vi "IV(H)_2devices_DC_vector_magnet_stable+sweep_BF_LD-400_K6221_K2182A_PK.vi"() -> ()   [LabVIEW 2016]
uses:
  Labview Drivers/Keithley 622x LV 2009/Keithley 622x.lvlib
  Labview Drivers/lake_shore_372/Lake Shore 372/Lake Shore 372.lvlib
panel:
  out "Still temperature (K)":dbl=0.747234 min=0.0 max=1000.0 step=1e-05 format="%^.5e"
  out "Still Output (%)":dbl=13.69 min=0.0 max=100.0 step=1e-05 format="%^.5e"
  out "Magnet temperature (K)":dbl=3.7122 min=0.0 max=1000.0 step=1e-05 format="%.5f"
  in  "From 5":dbl[](array[numeric])=[0.0] min=-3000.0 max=3000.0 format="%#.5f"
  in  "To 5":dbl[](array[numeric])=[0.0] min=-3000.0 max=3000.0 format="%#.5g"
  in  "Step 5":dbl[](array[numeric])=[0.001] min=-3000.0 max=3000.0 format="%.5e"
  in  "Still Heater Output (%)":dbl=13.69
  in  "Heater Range (0: Off)":u16(ring)=6 items=["Off", "31.6 uA", "100 uA", "316 uA", "1.00 mA", "3.16 mA", "10.0 mA", "31.6 mA", "100 mA"]
  in  "Output (0: sample heater)":u16(ring) items=["sample heater", "output 1 (warm-up heater) ", "output 2 (analog/still)"]
  in  "Rate(D) (0)":dbl min=0.0 max=2500.0 step=1.0 format="%.6f"
  in  "Reset(I) (20)":dbl=20.0 min=0.0 max=10000.0 step=1.0 format="%.6f"
  in  "Gain(P) (10.000)":dbl=10.0 min=0.001 max=1000.0 step=0.001 format="%.6f"
  out "Set Temperature (K)":dbl=0.9999999999999999 format="%#_13g"
  out "Delay timer (s)":i32=600
  in  "T settling delay (s)":i32=60
  out "Heater Output (%)":dbl=7.0 min=0.0 max=100.0 step=1e-05 format="%^.5e"
  out "Current Temperature (K)":dbl=1.00279 format="%#_13g"
  out "data 2":dbl[](array[numeric])=[0.0, 0.1539956170131437, 179.99925141305565, -5.8e-05, -0.000894677769, 15.42547877586207, 62218.001]
  out "File path 2":path=path "D:/Malli/GeTe/VNM519/027_VNM519_Dev1_DC_IV_baseT_OOP-Y-axis(250_to_-250mT)_1mT_steps_I16-19_V17-18_(K6221_12- K2182_4).dat"
  in  "Measure two devices?":bool
  in  "Number Averaging":i32=1
  in  "Tab Control":enum32{"Device 1", "Device 2"}(tab)
  out "V vs I":cluster{dbl, "Field Reading":dbl}[](graph)=[{0.0, "Field Reading"=-1.52268497e-07}, {2e-07, "Field Reading"=-7.97594228e-08}, {4e-07, "Field Reading"=-2.74494669e-08}, {6e-07, "Field Reading"=2.5999633e-07}, {8e-07, "Field Reading"=6.6863549e-07}, {1e-06, "Field Reading"=9.26042323e-07}, {1.2e-06, "Field Reading"=1.14823021e-06}, {1.4e-06, "Field Reading"=1.4843606e-06}, {1.6e-06, "Field Reading"=1.76714547e-06}, {1.8e-06, "Field Reading"=1.96654487e-06}, {2e-06, "Field Reading"=2.31562332e-06}, {2.2e-06, "Field Reading"=2.42801356e-06}, {2.4e-06, "Field Reading"=2.6657392e-06}, {2.6e-06, "Field Reading"=3.04123176e-06}, {2.8e-06, "Field Reading"=3.30122805e-06}, {3e-06, "Field Reading"=3.42190359e-06}, {3.2e-06, "Field Reading"=3.80050368e-06}, {3.4e-06, "Field Reading"=3.8305433e-06}, {3.6e-06, "Field Reading"=4.18790866e-06}, {3.8e-06, "Field Reading"=4.36969886e-06}, {4e-06, "Field Reading"=4.7099712e-06}, {4.2e-06, "Field Reading"=5.08080239e-06}, {4.4e-06, "Field Reading"=5.22633809e-06}, {4.6e-06, "Field Reading"=5.43764972e-06}, {4.8e-06, "Field Reading"=5.58784671e-06}, {5e-06, "Field Reading"=5.92760266e-06}, {5.2e-06, "Field Reading"=6.16066695e-06}, {5.4e-06, "Field Reading"=6.52631866e-06}, {5.6e-06, "Field Reading"=6.60711428e-06}, {5.8e-06, "Field Reading"=6.8862735e-06}, {6e-06, "Field Reading"=7.20945277e-06}, {6.2e-06, "Field Reading"=7.31976981e-06}, {6.4e-06, "Field Reading"=7.68645747e-06}, {6.6e-06, "Field Reading"=7.9987682e-06}, {6.8e-06, "Field Reading"=8.25462103e-06}, {7e-06, "Field Reading"=8.2913934e-06}, {7.2e-06, "Field Reading"=8.71400919e-06}, {7.4e-06, "Field Reading"=8.98850694e-06}, {7.6e-06, "Field Reading"=9.18531665e-06}, {7.8e-06, "Field Reading"=9.47948819e-06}, {8e-06, "Field Reading"=9.61984449e-06}, {8.2e-06, "Field Reading"=9.91195133e-06}, {8.4e-06, "Field Reading"=1.00347079e-05}, {8.6e-06, "Field Reading"=1.03490855e-05}, {8.8e-06, "Field Reading"=1.06489614e-05}, {9e-06, "Field Reading"=1.08991132e-05}, {9.2e-06, "Field Reading"=1.1134249e-05}, {9.4e-06, "Field Reading"=1.13165569e-05}, {9.6e-06, "Field Reading"=1.15257967e-05}, {9.8e-06, "Field Reading"=1.18443188e-05}, {1e-05, "Field Reading"=1.21214061e-05}, {1.02e-05, "Field Reading"=1.23254667e-05}, {1.04e-05, "Field Reading"=1.26320829e-05}, {1.06e-05, "Field Reading"=1.27895307e-05}, {1.08e-05, "Field Reading"=1.30749049e-05}, {1.1e-05, "Field Reading"=1.32494289e-05}, {1.12e-05, "Field Reading"=1.34664374e-05}, {1.14e-05, "Field Reading"=1.3915992e-05}, {1.16e-05, "Field Reading"=1.40470318e-05}, {1.18e-05, "Field Reading"=1.43101353e-05}, {1.2e-05, "Field Reading"=1.45571832e-05}, {1.22e-05, "Field Reading"=1.46328053e-05}, {1.24e-05, "Field Reading"=1.50393728e-05}, {1.26e-05, "Field Reading"=1.51921593e-05}, {1.28e-05, "Field Reading"=1.54972138e-05}, {1.3e-05, "Field Reading"=1.57333855e-05}, {1.32e-05, "Field Reading"=1.59866486e-05}, {1.34e-05, "Field Reading"=1.6305696e-05}, {1.36e-05, "Field Reading"=1.64346582e-05}, {1.38e-05, "Field Reading"=1.66801526e-05}, {1.4e-05, "Field Reading"=1.69613835e-05}, {1.42e-05, "Field Reading"=1.71208941e-05}, {1.44e-05, "Field Reading"=1.74218058e-05}, {1.46e-05, "Field Reading"=1.76522803e-05}, {1.48e-05, "Field Reading"=1.80106844e-05}, {1.5e-05, "Field Reading"=1.80904442e-05}, {1.52e-05, "Field Reading"=1.83623524e-05}, {1.54e-05, "Field Reading"=1.86627412e-05}, {1.56e-05, "Field Reading"=1.88631763e-05}, {1.58e-05, "Field Reading"=1.90320183e-05}, {1.6e-05, "Field Reading"=1.93800576e-05}, {1.62e-05, "Field Reading"=1.9578939e-05}, {1.64e-05, "Field Reading"=1.97788562e-05}, {1.66e-05, "Field Reading"=2.00880632e-05}, {1.68e-05, "Field Reading"=2.0350131e-05}, {1.7e-05, "Field Reading"=2.05593708e-05}, {1.72e-05, "Field Reading"=2.0896531e-05}, {1.74e-05, "Field Reading"=2.10658909e-05}, {1.76e-05, "Field Reading"=2.11917455e-05}, {1.78e-05, "Field Reading"=2.15387632e-05}, {1.8e-05, "Field Reading"=2.17775246e-05}, {1.82e-05, "Field Reading"=2.19841749e-05}, {1.84e-05, "Field Reading"=2.22824971e-05}, {1.86e-05, "Field Reading"=2.24321761e-05}, {1.88e-05, "Field Reading"=2.27020127e-05}, {1.9e-05, "Field Reading"=2.29822077e-05}, {1.92e-05, "Field Reading"=2.32157907e-05}, {1.94e-05, "Field Reading"=2.3448855e-05}, {1.96e-05, "Field Reading"=2.36135537e-05}, {1.98e-05, "Field Reading"=2.38725181e-05}, {2e-05, "Field Reading"=2.41837884e-05}, {2.02e-05, "Field Reading"=2.43945821e-05}, {2.04e-05, "Field Reading"=2.46193413e-05}, {2.06e-05, "Field Reading"=2.49093766e-05}, {2.08e-05, "Field Reading"=2.51222418e-05}, {2.1e-05, "Field Reading"=2.52900611e-05}, {2.12e-05, "Field Reading"=2.55407347e-05}, {2.14e-05, "Field Reading"=2.58758293e-05}, {2.16e-05, "Field Reading"=2.60860873e-05}, {2.18e-05, "Field Reading"=2.6178795e-05}, {2.2e-05, "Field Reading"=2.6620063e-05}, {2.22e-05, "Field Reading"=2.67676686e-05}, {2.24e-05, "Field Reading"=2.69230447e-05}, {2.26e-05, "Field Reading"=2.72975009e-05}, {2.28e-05, "Field Reading"=2.7582357e-05}, {2.3e-05, "Field Reading"=2.77507011e-05}, {2.32e-05, "Field Reading"=2.80096614e-05}, {2.34e-05, "Field Reading"=2.81696988e-05}, {2.36e-05, "Field Reading"=2.85907685e-05}, {2.38e-05, "Field Reading"=2.87735944e-05}, {2.4e-05, "Field Reading"=2.90294472e-05}, {2.42e-05, "Field Reading"=2.9178615e-05}, {2.44e-05, "Field Reading"=2.96002024e-05}, {2.46e-05, "Field Reading"=2.9786136e-05}, {2.48e-05, "Field Reading"=2.99565396e-05}, {2.6e-05, "Field Reading"=3.14186299e-05}, {2.7e-05, "Field Reading"=3.26751057e-05}, {2.8e-05, "Field Reading"=3.38378258e-05}, {2.9e-05, "Field Reading"=3.52035824e-05}, {3e-05, "Field Reading"=3.63435256e-05}, {3e-05, "Field Reading"=3.63673343e-05}, {1.501e-05, "Field Reading"=1.79573366e-05}, {2e-08, "Field Reading"=-3.87921991e-07}, {0.0, "Field Reading"=-3.45452353e-07}, {-2e-07, "Field Reading"=-3.83778479e-07}, {-4e-07, "Field Reading"=-4.92023888e-07}, {-6e-07, "Field Reading"=-7.5460964e-07}, {-8e-07, "Field Reading"=-1.24196958e-06}, {-1e-06, "Field Reading"=-1.538736e-06}, {-1.2e-06, "Field Reading"=-1.68893191e-06}, {-1.4e-06, "Field Reading"=-2.02972104e-06}, {-1.6e-06, "Field Reading"=-2.24103112e-06}, {-1.8e-06, "Field Reading"=-2.59114291e-06}, {-2e-06, "Field Reading"=-2.7993462e-06}, {-2.2e-06, "Field Reading"=-2.92209253e-06}, {-2.4e-06, "Field Reading"=-3.30068989e-06}, {-2.6e-06, "Field Reading"=-3.44466872e-06}, {-2.8e-06, "Field Reading"=-3.70673454e-06}, {-3e-06, "Field Reading"=-3.97190785e-06}, {-3.2e-06, "Field Reading"=-4.17493005e-06}, {-3.4e-06, "Field Reading"=-4.41472537e-06}, {-3.6e-06, "Field Reading"=-4.66177152e-06}, {-3.8e-06, "Field Reading"=-4.9191763e-06}, {-4e-06, "Field Reading"=-5.20920954e-06}, {-4.2e-06, "Field Reading"=-5.55465984e-06}, {-4.4e-06, "Field Reading"=-5.66652605e-06}, {-4.6e-06, "Field Reading"=-5.96691739e-06}, {-4.8e-06, "Field Reading"=-6.19013923e-06}, {-5e-06, "Field Reading"=-6.40818191e-06}, {-5.2e-06, "Field Reading"=-6.672842e-06}, {-5.4e-06, "Field Reading"=-6.9483736e-06}, {-5.6e-06, "Field Reading"=-7.18713312e-06}, {-5.8e-06, "Field Reading"=-7.36218605e-06}, {-6e-06, "Field Reading"=-7.68329416e-06}, {-6.2e-06, "Field Reading"=-7.86922612e-06}, {-6.4e-06, "Field Reading"=-8.26853861e-06}, {-6.6e-06, "Field Reading"=-8.30634649e-06}, {-6.8e-06, "Field Reading"=-8.59586168e-06}, {-7e-06, "Field Reading"=-9.00657456e-06}, {-7.2e-06, "Field Reading"=-9.14951953e-06}, {-7.4e-06, "Field Reading"=-9.39708366e-06}, {-7.6e-06, "Field Reading"=-9.56643916e-06}, {-7.8e-06, "Field Reading"=-9.81970027e-06}, {-8e-06, "Field Reading"=-1.00263489e-05}, {-8.2e-06, "Field Reading"=-1.02837565e-05}, {-8.4e-06, "Field Reading"=-1.06437086e-05}, {-8.6e-06, "Field Reading"=-1.07623114e-05}, {-8.8e-06, "Field Reading"=-1.09855426e-05}, {-9e-06, "Field Reading"=-1.11694032e-05}, {-9.2e-06, "Field Reading"=-1.15034596e-05}, {-9.4e-06, "Field Reading"=-1.17209848e-05}, {-9.6e-06, "Field Reading"=-1.19462748e-05}, {-9.8e-06, "Field Reading"=-1.21871062e-05}, {-1e-05, "Field Reading"=-1.24362242e-05}, {-1.02e-05, "Field Reading"=-1.26667036e-05}, {-1.04e-05, "Field Reading"=-1.30364964e-05}, {-1.06e-05, "Field Reading"=-1.32317511e-05}, {-1.08e-05, "Field Reading"=-1.35373222e-05}, {-1.1e-05, "Field Reading"=-1.37237724e-05}, {-1.12e-05, "Field Reading"=-1.40371123e-05}, {-1.14e-05, "Field Reading"=-1.42893266e-05}, {-1.16e-05, "Field Reading"=-1.43830695e-05}, {-1.18e-05, "Field Reading"=-1.46358129e-05}, {-1.2e-05, "Field Reading"=-1.50543024e-05}, {-1.22e-05, "Field Reading"=-1.51656546e-05}, {-1.24e-05, "Field Reading"=-1.54468836e-05}, {-1.26e-05, "Field Reading"=-1.56442061e-05}, {-1.28e-05, "Field Reading"=-1.580735e-05}, {-1.3e-05, "Field Reading"=-1.61113673e-05}, {-1.32e-05, "Field Reading"=-1.62418839e-05}, {-1.34e-05, "Field Reading"=-1.6634983e-05}, {-1.36e-05, "Field Reading"=-1.68178077e-05}, {-1.38e-05, "Field Reading"=-1.69198374e-05}, {-1.4e-05, "Field Reading"=-1.7212986e-05}, {-1.42e-05, "Field Reading"=-1.74341367e-05}, {-1.44e-05, "Field Reading"=-1.77231346e-05}, {-1.46e-05, "Field Reading"=-1.78510457e-05}, {-1.48e-05, "Field Reading"=-1.81830304e-05}, {-1.5e-05, "Field Reading"=-1.83668909e-05}, {-1.52e-05, "Field Reading"=-1.86812606e-05}, {-1.54e-05, "Field Reading"=-1.87755215e-05}, {-1.56e-05, "Field Reading"=-1.91867473e-05}, {-1.58e-05, "Field Reading"=-1.92447572e-05}, {-1.6e-05, "Field Reading"=-1.95373802e-05}, {-1.62e-05, "Field Reading"=-1.98776515e-05}, {-1.64e-05, "Field Reading"=-2.01619878e-05}, {-1.66e-05, "Field Reading"=-2.03448124e-05}, {-1.68e-05, "Field Reading"=-2.05985916e-05}, {-1.7e-05, "Field Reading"=-2.09740769e-05}, {-1.72e-05, "Field Reading"=-2.10243148e-05}, {-1.74e-05, "Field Reading"=-2.14578111e-05}, {-1.76e-05, "Field Reading"=-2.17752926e-05}, {-1.78e-05, "Field Reading"=-2.20503063e-05}, {-1.8e-05, "Field Reading"=-2.21507822e-05}, {-1.82e-05, "Field Reading"=-2.23900597e-05}, {-1.84e-05, "Field Reading"=-2.26723233e-05}, {-1.86e-05, "Field Reading"=-2.28976171e-05}, {-1.88e-05, "Field Reading"=-2.31016762e-05}, {-1.9e-05, "Field Reading"=-2.34289957e-05}, {-1.92e-05, "Field Reading"=-2.37117782e-05}, {-1.94e-05, "Field Reading"=-2.40458343e-05}, {-1.96e-05, "Field Reading"=-2.40541191e-05}, {-1.98e-05, "Field Reading"=-2.44544686e-05}, {-2e-05, "Field Reading"=-2.46621531e-05}, {-2.02e-05, "Field Reading"=-2.49703066e-05}, {-2.04e-05, "Field Reading"=-2.5097714e-05}, {-2.06e-05, "Field Reading"=-2.54835617e-05}, {-2.08e-05, "Field Reading"=-2.55648796e-05}, {-2.1e-05, "Field Reading"=-2.58497336e-05}, {-2.12e-05, "Field Reading"=-2.60413627e-05}, {-2.14e-05, "Field Reading"=-2.64365387e-05}, {-2.16e-05, "Field Reading"=-2.67032657e-05}, {-2.18e-05, "Field Reading"=-2.68964486e-05}, {-2.2e-05, "Field Reading"=-2.71341792e-05}, {-2.22e-05, "Field Reading"=-2.72719451e-05}, {-2.24e-05, "Field Reading"=-2.75303855e-05}, {-2.26e-05, "Field Reading"=-2.79266128e-05}, {-2.28e-05, "Field Reading"=-2.81301542e-05}, {-2.3e-05, "Field Reading"=-2.83901486e-05}, {-2.32e-05, "Field Reading"=-2.84232953e-05}, {-2.34e-05, "Field Reading"=-2.87630526e-05}, {-2.36e-05, "Field Reading"=-2.91333634e-05}, {-2.38e-05, "Field Reading"=-2.9317224e-05}, {-2.4e-05, "Field Reading"=-2.96481828e-05}, {-2.42e-05, "Field Reading"=-2.98304898e-05}, {-2.44e-05, "Field Reading"=-2.99692916e-05}, {-2.46e-05, "Field Reading"=-3.02660647e-05}, {-2.48e-05, "Field Reading"=-3.04944663e-05}, {-2.6e-05, "Field Reading"=-3.20653099e-05}, {-2.7e-05, "Field Reading"=-3.32523697e-05}, {-2.8e-05, "Field Reading"=-3.44534201e-05}, {-2.9e-05, "Field Reading"=-3.56938321e-05}, {-3e-05, "Field Reading"=-3.69958442e-05}, {-3e-05, "Field Reading"=-3.70222579e-05}, {-1.501e-05, "Field Reading"=-1.84243803e-05}, {-2e-08, "Field Reading"=-2.59477872e-07}]
  in  "File name 1":string="011_31-05-2022_DevB4_DC_IV(H)_baseT_[5_to-5mT]_30uT_steps_(0_deg)_I_10-36_V_12-37_100nA_steps"
  in  "From 3":dbl[](array[numeric])=[0.0, 2e-05, 0.0, -2e-05] min=-3000.0 max=3000.0 format="%.1e"
  in  "To 3":dbl[](array[numeric])=[2e-05, 0.0, -2e-05, 0.0] min=-3000.0 max=3000.0 format="%.1e"
  in  "Step 3":dbl[](array[numeric])=[2e-08, 9.99e-06, 2e-08, 9.99e-06] min=-3000.0 max=3000.0 format="%.1e"
  in  "Current source K6221 VISA Device 1":refnum<visa-resource-name>="GPIB0::13::INSTR"
  in  "Nanovoltmeter 2182a VISA Device1":refnum<visa-resource-name>="GPIB0::7::INSTR"
  in  "wait (ms)":u32=50
  in  "Set Compliance voltage (V)":dbl=2.0 min=0.0 step=0.1 format="%_3f"
  out "Resistance (ohm)":dbl=12.9738936 format="%#_13g"
  out "Time (s)":dbl=151861.951 format="%#_13g"
  out "Iset (A)":dbl=-2e-08
  out "Vmeas (V)":dbl=-2.59477872e-07
  in  "File name 2":string="040_31-05-2023_DevB3_DC_IV(A)_baseT_12mT_(0-360deg)_5deg_steps_I_10-38_V_12-31_"
  in  "Current source K6221 VISA Device 2":refnum<visa-resource-name>="GPIB0::13::INSTR"
  in  "Nanovoltmeter 2182a VISA Device 2":refnum<visa-resource-name>="GPIB0::7::INSTR"
  in  "Set Compliance voltage (V) 2":dbl=2.0 min=0.0 step=0.1 format="%_3f"
  in  "wait (ms) 2":u32=50
  in  "To 4":dbl[](array[numeric])=[1e-05, 3e-05, -1e-05, -0.0001, 0.0] min=-3000.0 max=3000.0 format="%.1e"
  in  "From 4":dbl[](array[numeric])=[0.0, 1.1e-05, 3e-05, 0.0, -0.0001] min=-3000.0 max=3000.0 format="%.1e"
  in  "Step 4":dbl[](array[numeric])=[2e-07, 1e-06, 0.0, 5e-07, 9.9e-05] min=-3000.0 max=3000.0 format="%.1e"
  out "V vs I 2":cluster{dbl, "Field Reading":dbl}[](graph)=[{0.0, "Field Reading"=1.05982577e-07}, {5e-07, "Field Reading"=1.23902621e-07}, {1e-06, "Field Reading"=4.09598972e-08}, {1.5e-06, "Field Reading"=7.78233302e-08}, {2e-06, "Field Reading"=7.52633791e-08}, {2.5e-06, "Field Reading"=9.9839001e-08}, {3e-06, "Field Reading"=6.70715052e-08}, {3.5e-06, "Field Reading"=6.34878296e-08}, {4e-06, "Field Reading"=1.95069789e-07}, {4.5e-06, "Field Reading"=1.48733775e-06}, {5e-06, "Field Reading"=3.68225755e-06}, {5.5e-06, "Field Reading"=7.0056209e-06}, {6e-06, "Field Reading"=1.131355e-05}, {6.5e-06, "Field Reading"=1.67191983e-05}, {7e-06, "Field Reading"=2.2852904e-05}, {7.5e-06, "Field Reading"=2.94079847e-05}, {8e-06, "Field Reading"=3.63951874e-05}, {8.5e-06, "Field Reading"=4.35057808e-05}, {9e-06, "Field Reading"=5.09056291e-05}, {9.5e-06, "Field Reading"=5.82773365e-05}, {1e-05, "Field Reading"=6.58016184e-05}, {1.05e-05, "Field Reading"=7.33770992e-05}, {1.1e-05, "Field Reading"=8.09648681e-05}, {1.15e-05, "Field Reading"=8.87364392e-05}, {1.2e-05, "Field Reading"=9.64209746e-05}, {1.25e-05, "Field Reading"=0.000104230437}, {1.3e-05, "Field Reading"=0.000112046003}, {1.35e-05, "Field Reading"=0.000119815015}, {1.4e-05, "Field Reading"=0.000127742783}, {1.45e-05, "Field Reading"=0.000135573235}, {1.5e-05, "Field Reading"=0.000143516327}, {1.55e-05, "Field Reading"=0.000151494156}, {1.6e-05, "Field Reading"=0.000159501242}, {1.65e-05, "Field Reading"=0.000167343466}, {1.7e-05, "Field Reading"=0.000175483152}, {1.75e-05, "Field Reading"=0.000183456446}, {1.8e-05, "Field Reading"=0.000191661699}, {1.85e-05, "Field Reading"=0.000199612466}, {1.9e-05, "Field Reading"=0.000207719848}, {1.95e-05, "Field Reading"=0.000215802195}, {2e-05, "Field Reading"=0.00022388403}, {2.05e-05, "Field Reading"=0.000232062763}, {2.1e-05, "Field Reading"=0.000240102107}, {2.15e-05, "Field Reading"=0.000247269011}, {2.2e-05, "Field Reading"=0.000255929973}, {2.25e-05, "Field Reading"=0.000264142372}, {2.3e-05, "Field Reading"=0.000272170452}, {2.35e-05, "Field Reading"=0.000280406012}, {2.4e-05, "Field Reading"=0.000288539055}, {2.45e-05, "Field Reading"=0.000296639977}, {2.5e-05, "Field Reading"=0.000304956829}, {2.55e-05, "Field Reading"=0.000312984916}, {2.6e-05, "Field Reading"=0.000321277684}, {2.65e-05, "Field Reading"=0.000329427113}, {2.7e-05, "Field Reading"=0.00033774076}, {2.75e-05, "Field Reading"=0.000346032008}, {2.8e-05, "Field Reading"=0.000354167609}, {2.85e-05, "Field Reading"=0.000362498087}, {2.9e-05, "Field Reading"=0.000370754002}, {2.95e-05, "Field Reading"=0.000379070387}, {3e-05, "Field Reading"=0.000387405662}, {3.05e-05, "Field Reading"=0.000395624202}, {3.1e-05, "Field Reading"=0.000403926088}, {3.15e-05, "Field Reading"=0.00041243339}, {3.2e-05, "Field Reading"=0.000420845302}, {3.25e-05, "Field Reading"=0.000429363875}, {3.3e-05, "Field Reading"=0.000437565523}, {3.35e-05, "Field Reading"=0.000446109155}, {3.4e-05, "Field Reading"=0.000454533008}, {3.45e-05, "Field Reading"=0.000463127356}, {3.5e-05, "Field Reading"=0.000471630056}, {3.55e-05, "Field Reading"=0.000479936662}, {3.6e-05, "Field Reading"=0.000488525981}, {3.65e-05, "Field Reading"=0.000497198664}, {3.7e-05, "Field Reading"=0.000505853053}, {3.75e-05, "Field Reading"=0.000514436643}, {3.8e-05, "Field Reading"=0.000522915273}, {3.85e-05, "Field Reading"=0.000531648928}, {3.9e-05, "Field Reading"=0.000540244293}, {3.95e-05, "Field Reading"=0.000548950249}, {4e-05, "Field Reading"=0.000557677924}, {4.05e-05, "Field Reading"=0.000566248716}, {4.1e-05, "Field Reading"=0.000574937679}, {4.15e-05, "Field Reading"=0.000583695347}, {4.2e-05, "Field Reading"=0.000592494999}, {4.25e-05, "Field Reading"=0.000601192661}, {4.3e-05, "Field Reading"=0.000609976951}, {4.35e-05, "Field Reading"=0.000618619419}, {4.4e-05, "Field Reading"=0.000627518275}, {4.45e-05, "Field Reading"=0.000636379362}, {4.5e-05, "Field Reading"=0.000644912509}, {4.55e-05, "Field Reading"=0.00065393999}, {4.6e-05, "Field Reading"=0.000662870466}, {4.65e-05, "Field Reading"=0.000671738209}, {4.7e-05, "Field Reading"=0.000680896763}, {4.75e-05, "Field Reading"=0.000689596876}, {4.8e-05, "Field Reading"=0.000698582898}, {4.85e-05, "Field Reading"=0.000707876118}, {4.9e-05, "Field Reading"=0.00071700519}, {4.95e-05, "Field Reading"=0.00072625694}, {5e-05, "Field Reading"=0.000735252693}, {5.05e-05, "Field Reading"=0.000744563505}, {5.1e-05, "Field Reading"=0.000753877714}, {5.15e-05, "Field Reading"=0.000763235462}, {5.2e-05, "Field Reading"=0.000772666405}, {5.25e-05, "Field Reading"=0.000781939653}, {5.3e-05, "Field Reading"=0.00079146705}, {5.35e-05, "Field Reading"=0.000801081283}, {5.4e-05, "Field Reading"=0.000810671964}, {5.45e-05, "Field Reading"=0.000820330099}, {5.5e-05, "Field Reading"=0.000830001161}, {5.55e-05, "Field Reading"=0.000839830429}, {5.6e-05, "Field Reading"=0.000849894446}, {5.65e-05, "Field Reading"=0.000859963842}, {5.7e-05, "Field Reading"=0.00087027569}, {5.75e-05, "Field Reading"=0.000880684023}, {5.8e-05, "Field Reading"=0.000891300225}, {5.85e-05, "Field Reading"=0.000901884572}, {5.9e-05, "Field Reading"=0.00091264413}, {5.95e-05, "Field Reading"=0.000923292586}, {6e-05, "Field Reading"=0.000933904184}, {6.05e-05, "Field Reading"=0.000944740541}, {6.1e-05, "Field Reading"=0.000955724863}, {6.15e-05, "Field Reading"=0.000966541693}, {6.2e-05, "Field Reading"=0.000977790203}, {6.25e-05, "Field Reading"=0.0009887668}, {6.3e-05, "Field Reading"=0.00100003886}, {6.35e-05, "Field Reading"=0.00101126331}, {6.4e-05, "Field Reading"=0.00102284095}, {6.45e-05, "Field Reading"=0.00103437413}, {6.5e-05, "Field Reading"=0.00104578697}, {6.55e-05, "Field Reading"=0.00105781627}, {6.6e-05, "Field Reading"=0.00106970781}, {6.65e-05, "Field Reading"=0.00108158658}, {6.7e-05, "Field Reading"=0.00109345152}, {6.75e-05, "Field Reading"=0.00110520407}, {6.8e-05, "Field Reading"=0.00111705365}, {6.85e-05, "Field Reading"=0.00112896007}, {6.9e-05, "Field Reading"=0.00114097245}, {6.95e-05, "Field Reading"=0.00115300225}, {7e-05, "Field Reading"=0.00116490713}, {7.05e-05, "Field Reading"=0.00117701585}, {7.1e-05, "Field Reading"=0.0011890902}, {7.15e-05, "Field Reading"=0.00120116737}, {7.2e-05, "Field Reading"=0.00121302054}, {7.25e-05, "Field Reading"=0.00122527818}, {7.3e-05, "Field Reading"=0.00123750597}, {7.35e-05, "Field Reading"=0.00124952144}, {7.4e-05, "Field Reading"=0.00126179393}, {7.45e-05, "Field Reading"=0.00127385138}, {7.5e-05, "Field Reading"=0.00128607011}, {7.55e-05, "Field Reading"=0.00129831901}, {7.6e-05, "Field Reading"=0.00131059815}, {7.65e-05, "Field Reading"=0.00132285322}, {7.7e-05, "Field Reading"=0.00133496366}, {7.75e-05, "Field Reading"=0.00134726123}, {7.8e-05, "Field Reading"=0.00135956111}, {7.85e-05, "Field Reading"=0.00137195033}, {7.9e-05, "Field Reading"=0.00138423407}, {7.95e-05, "Field Reading"=0.00139647286}, {8e-05, "Field Reading"=0.00140887898}, {8.05e-05, "Field Reading"=0.00142125669}, {8.1e-05, "Field Reading"=0.00143369762}, {8.15e-05, "Field Reading"=0.00144604179}, {8.2e-05, "Field Reading"=0.00145820055}, {8.25e-05, "Field Reading"=0.0014708299}, {8.3e-05, "Field Reading"=0.001483259}, {8.35e-05, "Field Reading"=0.00149571273}, {8.4e-05, "Field Reading"=0.00150827449}, {8.45e-05, "Field Reading"=0.00152058173}, {8.5e-05, "Field Reading"=0.00153315169}, {8.55e-05, "Field Reading"=0.00154567403}, {8.6e-05, "Field Reading"=0.00155821094}, {8.65e-05, "Field Reading"=0.00157085359}, {8.7e-05, "Field Reading"=0.00158327521}, {8.75e-05, "Field Reading"=0.00159591991}, {8.8e-05, "Field Reading"=0.00160856665}, {8.85e-05, "Field Reading"=0.00162121374}, {8.9e-05, "Field Reading"=0.00163385997}, {8.95e-05, "Field Reading"=0.00164634288}, {9e-05, "Field Reading"=0.00165906267}, {9.05e-05, "Field Reading"=0.00167177904}, {9.1e-05, "Field Reading"=0.00168450438}, {9.15e-05, "Field Reading"=0.00169730779}, {9.2e-05, "Field Reading"=0.00170982705}, {9.25e-05, "Field Reading"=0.00172262613}, {9.3e-05, "Field Reading"=0.00173539114}, {9.35e-05, "Field Reading"=0.00174822988}, {9.4e-05, "Field Reading"=0.00176107221}, {9.45e-05, "Field Reading"=0.00177372408}, {9.5e-05, "Field Reading"=0.00178659463}, {9.55e-05, "Field Reading"=0.00179942159}, {9.6e-05, "Field Reading"=0.00181213335}, {9.65e-05, "Field Reading"=0.00182507038}, {9.7e-05, "Field Reading"=0.00183795264}, {9.75e-05, "Field Reading"=0.00185079437}, {9.8e-05, "Field Reading"=0.0018638159}, {9.85e-05, "Field Reading"=0.00187644421}, {9.9e-05, "Field Reading"=0.0018893681}, {9.95e-05, "Field Reading"=0.001902598}, {0.0001, "Field Reading"=0.00191566643}, {0.0001, "Field Reading"=0.00191578214}, {1e-06, "Field Reading"=1.04959382e-07}, {0.0, "Field Reading"=6.2978119e-08}, {-5e-07, "Field Reading"=7.37299411e-08}, {-1e-06, "Field Reading"=7.32183306e-08}, {-1.5e-06, "Field Reading"=9.8305911e-08}, {-2e-06, "Field Reading"=9.8305911e-08}, {-2.5e-06, "Field Reading"=-9.212857e-09}, {-3e-06, "Field Reading"=7.52657514e-08}, {-3.5e-06, "Field Reading"=-2.29881222e-07}, {-4e-06, "Field Reading"=-9.66638942e-07}, {-4.5e-06, "Field Reading"=-2.71867509e-06}, {-5e-06, "Field Reading"=-5.44042382e-06}, {-5.5e-06, "Field Reading"=-9.24299578e-06}, {-6e-06, "Field Reading"=-1.39195329e-05}, {-6.5e-06, "Field Reading"=-1.93947706e-05}, {-7e-06, "Field Reading"=-2.53845658e-05}, {-7.5e-06, "Field Reading"=-3.17772987e-05}, {-8e-06, "Field Reading"=-3.85647725e-05}, {-8.5e-06, "Field Reading"=-4.54935603e-05}, {-9e-06, "Field Reading"=-5.25713378e-05}, {-9.5e-06, "Field Reading"=-5.9848778e-05}, {-1e-05, "Field Reading"=-6.72593486e-05}, {-1.05e-05, "Field Reading"=-7.46959979e-05}, {-1.1e-05, "Field Reading"=-8.22145956e-05}, {-1.15e-05, "Field Reading"=-8.98888387e-05}, {-1.2e-05, "Field Reading"=-9.7508345e-05}, {-1.25e-05, "Field Reading"=-0.000105279358}, {-1.3e-05, "Field Reading"=-0.000112994564}, {-1.35e-05, "Field Reading"=-0.000120810121}, {-1.4e-05, "Field Reading"=-0.000128620045}, {-1.45e-05, "Field Reading"=-0.00013646688}, {-1.5e-05, "Field Reading"=-0.000144369477}, {-1.55e-05, "Field Reading"=-0.000152356042}, {-1.6e-05, "Field Reading"=-0.00016028334}, {-1.65e-05, "Field Reading"=-0.000168222807}, {-1.7e-05, "Field Reading"=-0.000176283573}, {-1.75e-05, "Field Reading"=-0.000184271677}, {-1.8e-05, "Field Reading"=-0.000192294085}, {-1.85e-05, "Field Reading"=-0.000200345666}, {-1.9e-05, "Field Reading"=-0.00020833633}, {-1.95e-05, "Field Reading"=-0.000216423693}, {-2e-05, "Field Reading"=-0.000224573584}, {-2.05e-05, "Field Reading"=-0.000232658964}, {-2.1e-05, "Field Reading"=-0.000240789835}, {-2.15e-05, "Field Reading"=-0.00024942458}, {-2.2e-05, "Field Reading"=-0.000257524758}, {-2.25e-05, "Field Reading"=-0.000265682837}, {-2.3e-05, "Field Reading"=-0.000273921299}, {-2.35e-05, "Field Reading"=-0.000281918732}, {-2.4e-05, "Field Reading"=-0.000290019983}, {-2.45e-05, "Field Reading"=-0.000298346441}, {-2.5e-05, "Field Reading"=-0.000306562888}, {-2.55e-05, "Field Reading"=-0.000314745032}, {-2.6e-05, "Field Reading"=-0.000322866101}, {-2.65e-05, "Field Reading"=-0.000331147056}, {-2.7e-05, "Field Reading"=-0.000339239598}, {-2.75e-05, "Field Reading"=-0.000347604575}, {-2.8e-05, "Field Reading"=-0.000355902938}, {-2.85e-05, "Field Reading"=-0.000364053667}, {-2.9e-05, "Field Reading"=-0.000372274716}, {-2.95e-05, "Field Reading"=-0.000380721042}, {-3e-05, "Field Reading"=-0.000389052226}, {-3.05e-05, "Field Reading"=-0.000397248701}, {-3.1e-05, "Field Reading"=-0.000405627052}, {-3.15e-05, "Field Reading"=-0.000414022694}, {-3.2e-05, "Field Reading"=-0.000422452566}, {-3.25e-05, "Field Reading"=-0.000430871246}, {-3.3e-05, "Field Reading"=-0.000439115251}, {-3.35e-05, "Field Reading"=-0.000447710054}, {-3.4e-05, "Field Reading"=-0.000456261339}, {-3.45e-05, "Field Reading"=-0.000464751635}, {-3.5e-05, "Field Reading"=-0.000473286534}, {-3.55e-05, "Field Reading"=-0.00048171494}, {-3.6e-05, "Field Reading"=-0.000490283148}, {-3.65e-05, "Field Reading"=-0.000498827776}, {-3.7e-05, "Field Reading"=-0.000507439986}, {-3.75e-05, "Field Reading"=-0.000516045781}, {-3.8e-05, "Field Reading"=-0.0005246155}, {-3.85e-05, "Field Reading"=-0.000533221482}, {-3.9e-05, "Field Reading"=-0.000541909479}, {-3.95e-05, "Field Reading"=-0.000550577507}, {-4e-05, "Field Reading"=-0.000559311386}, {-4.05e-05, "Field Reading"=-0.000567846814}, {-4.1e-05, "Field Reading"=-0.00057664276}, {-4.15e-05, "Field Reading"=-0.000585338952}, {-4.2e-05, "Field Reading"=-0.000594088391}, {-4.25e-05, "Field Reading"=-0.00060273111}, {-4.3e-05, "Field Reading"=-0.000611546081}, {-4.35e-05, "Field Reading"=-0.00062030934}, {-4.4e-05, "Field Reading"=-0.000629159621}, {-4.45e-05, "Field Reading"=-0.0006379664}, {-4.5e-05, "Field Reading"=-0.000646666684}, {-4.55e-05, "Field Reading"=-0.000655509687}, {-4.6e-05, "Field Reading"=-0.000664396847}, {-4.65e-05, "Field Reading"=-0.000673287336}, {-4.7e-05, "Field Reading"=-0.000682299425}, {-4.75e-05, "Field Reading"=-0.000691233691}, {-4.8e-05, "Field Reading"=-0.000700295086}, {-4.85e-05, "Field Reading"=-0.00070939524}, {-4.9e-05, "Field Reading"=-0.000718437027}, {-4.95e-05, "Field Reading"=-0.000727632333}, {-5e-05, "Field Reading"=-0.000736695622}, {-5.05e-05, "Field Reading"=-0.000746025716}, {-5.1e-05, "Field Reading"=-0.000755243116}, {-5.15e-05, "Field Reading"=-0.000764786655}, {-5.2e-05, "Field Reading"=-0.000774240444}, {-5.25e-05, "Field Reading"=-0.000783658543}, {-5.3e-05, "Field Reading"=-0.000793342878}, {-5.35e-05, "Field Reading"=-0.000803049948}, {-5.4e-05, "Field Reading"=-0.000812865349}, {-5.45e-05, "Field Reading"=-0.000822671023}, {-5.5e-05, "Field Reading"=-0.000832792343}, {-5.55e-05, "Field Reading"=-0.000842879097}, {-5.6e-05, "Field Reading"=-0.000853268375}, {-5.65e-05, "Field Reading"=-0.000863553781}, {-5.7e-05, "Field Reading"=-0.00087382946}, {-5.75e-05, "Field Reading"=-0.000884019633}, {-5.8e-05, "Field Reading"=-0.000894677769}]
  out "Vmeas (V) 2":dbl=-0.000894677769
  out "Resistance (ohm) 2":dbl=15.42547877586207 format="%#_13g"
  out "Iset (A) 2":dbl=-5.8e-05
  out "Sweeping Magnetic Field magnitude(T)":dbl=284.9997059221995 format="%#_13g"
  out "Stable Magnetic Field magnitude (T)":dbl=0.11799861557435369 format="%#_13g"
  in  "From 2":dbl[](array[numeric])=[0.005] min=-3000.0 max=3000.0 format="%#.5f"
  in  "To 2":dbl[](array[numeric])=[-0.005] min=-3000.0 max=3000.0 format="%#.5g"
  in  "Step 2":dbl[](array[numeric])=[3e-05] min=-3000.0 max=3000.0 format="%.5e"
  in  "Wait time after each sweep(min)":dbl=0.1 format="%#_13g"
  in  "Sweep Field ramp rate (T/min)":string="0.0005"
  in  "Stable Field ramp rate (T/min)":string="0.0005"
  in  "Magnet IP Address \n(Stable field)":string="169.254.207.70"
  in  "Magnet IP Address\n(Sweeping  field)":string="169.254.67.34"
  in  "Magnetic field stabilization time (s)":dbl=1.0 format="%#_13g"
  in  "Step":dbl[](array[numeric])=[0.001] min=-3000.0 max=3000.0 format="%.4g"
  in  "To":dbl[](array[numeric])=[0.0] min=-3000.0 max=3000.0 format="%.4f"
  in  "From":dbl[](array[numeric])=[0.0] min=-3000.0 max=3000.0 format="%.4f"
  in  "Folder":path=path "D:/Pranava/Data/PtTe2/31-05-2022/001/Round8_IP/after warmup"
  out "data":dbl[](array[numeric])=[1.00279, 0.11799861557435369, 284.9997059221995, -2e-08, -2.59477872e-07, 12.9738936, 151861.951]
  out "File path 1":path=path "D:/Pranava/Data/PtTe2/31-05-2022/001/Round8_IP/after warmup/011_31-05-2022_DevB4_DC_IV(H)_baseT_[5_to-5mT]_30uT_steps_(0_deg)_I_10-36_V_12-37_100nA_steps.dat"
  # "11.5% corresponds to 7mW\n13.69% corresponds to 10mW\nSet to 0 if you want to use at 1K"
  # "[Must be less than 0.05]"
  # "It is important that there is enough time for the magnet to cool down after each sweep (Typically 15-20 min)"
  # "Configure Temperature (K)"
  # "Configure Stable Field (T)"
  # "Configure Sweeping Field(T)"
  # "Z-Axis: In-plane (90 deg)\nY-axis: Out-of-plane (0 deg)"
  # ".dat"
  # "Configure current sweep 1 (A)"
  # ".dat"
  # "Configure current sweep 2 (A)"
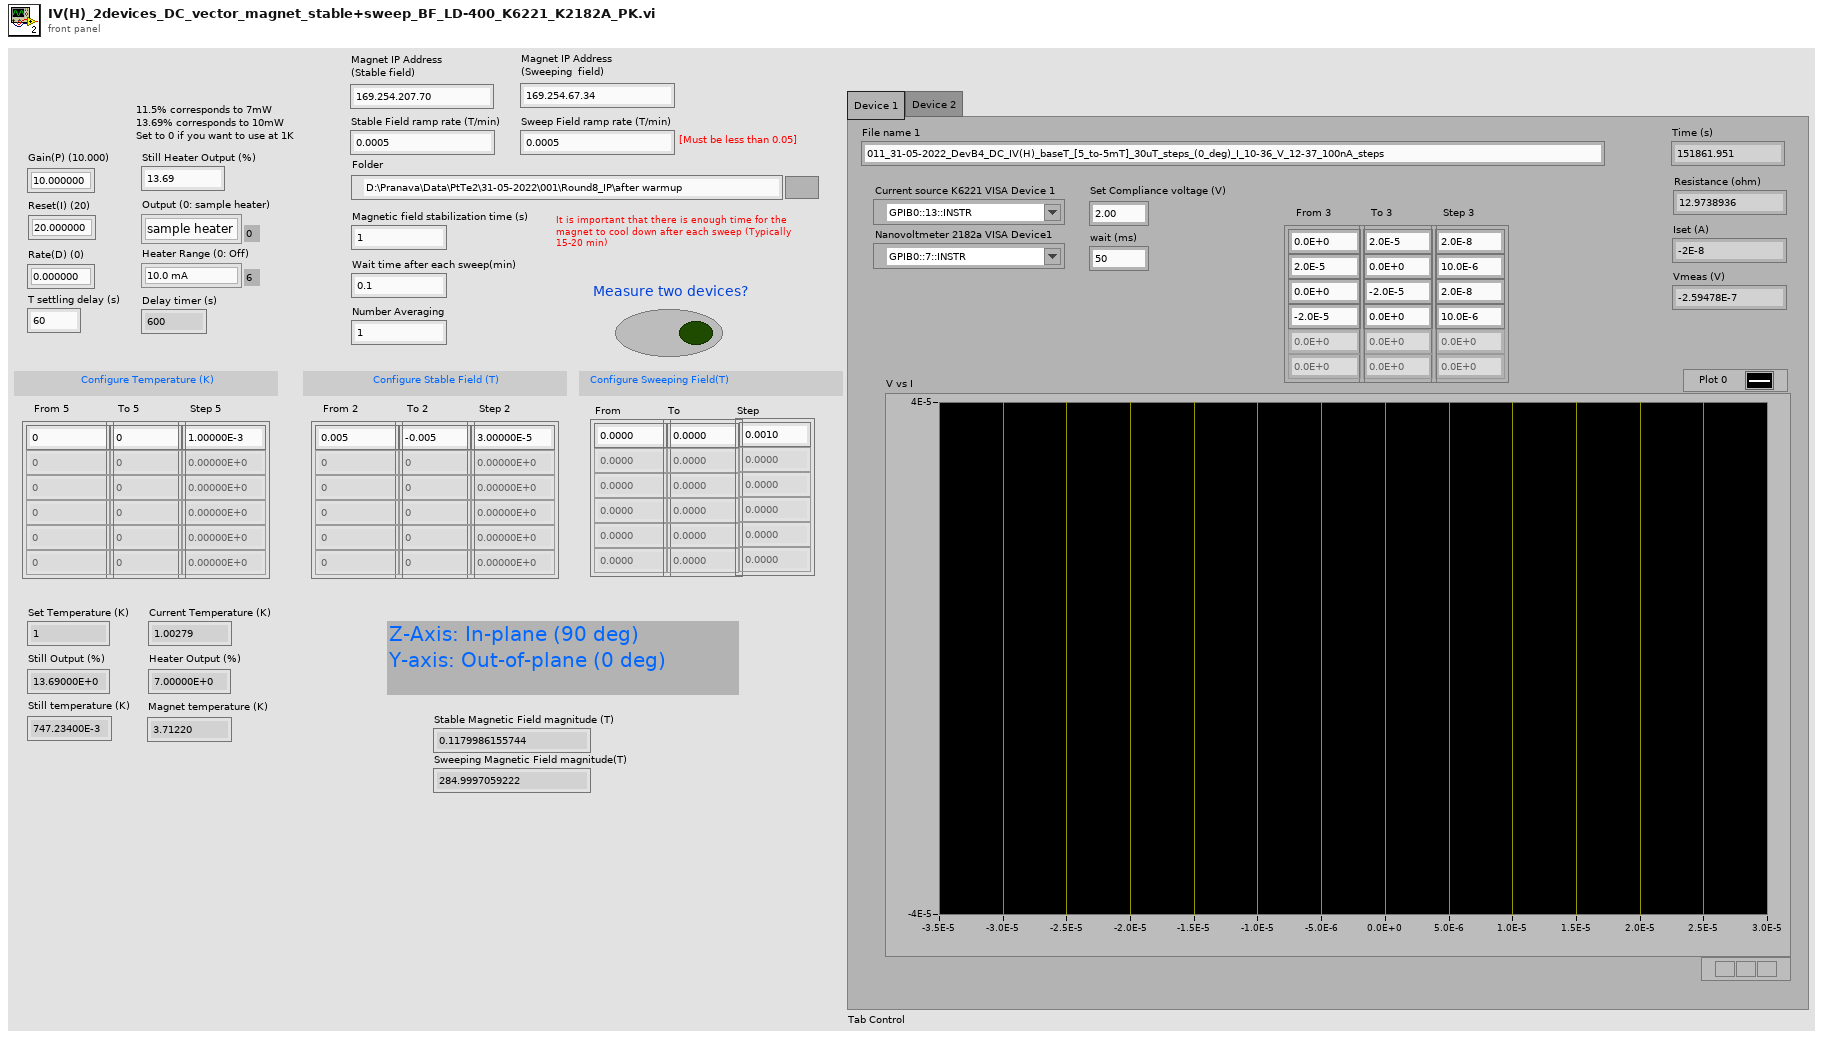
[diagram p1: front panel]
types:
  T1 = enum16{"open", "replace", "create", "open or create", "replace or create", "replace or create with confirmation"}
  T2 = typedef "Keithley 622x.lvlib/KE622x -- Current Level.ctl" = dbl
  T3 = cluster{"Average value":dbl, "Average value":dbl}
  T4 = cluster{"Average value":dbl, "Average value":dbl}[]
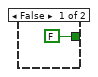
[diagram p2: hidden frame]
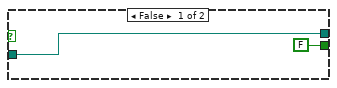
[diagram p3: hidden frame]
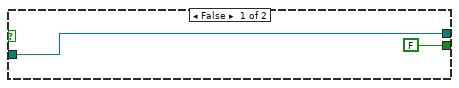
[diagram p5: hidden frame]
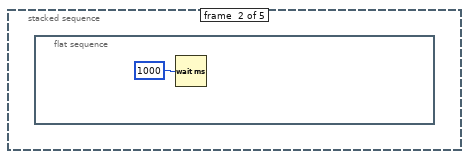
[diagram p6: hidden frame]
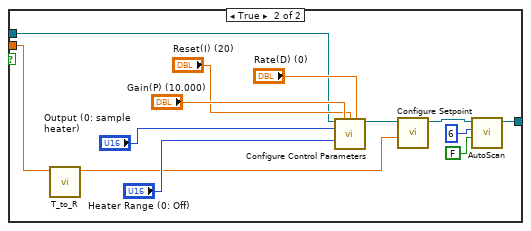
[diagram p9: hidden frame]
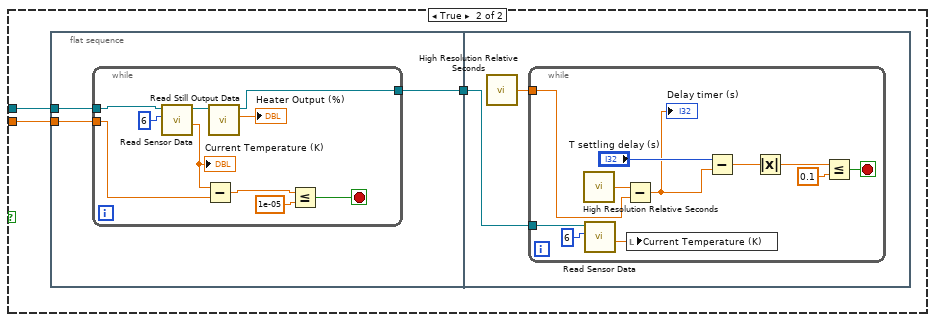
[diagram p10: hidden frame]
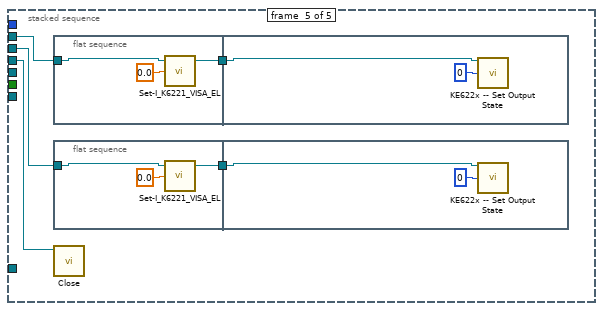
[diagram p13: hidden frame]
diagram:
  n1 = call "430_TCP_Open.vi"("IP Address"="Magnet IP Address \n(Stable field)", "TCP Port"=7180) -> ("connection ID"=w7:refnum<k5>)  [unwired: 4 in, 2 out]
  n2 = call "430_TCP_Open.vi"("IP Address"="Magnet IP Address\n(Sweeping  field)", "TCP Port"=7180) -> ("connection ID"=w12:refnum<k5>)  [unwired: 4 in, 2 out]
  n3 = Tick Count (ms)() -> (millisecond timer value=w11:u32)
  n4 = stacked-sequence {
    tunnel: w12 -> [w31 _ _ w139 _]
    tunnel: w11 -> [_ _ _ w166 _]
    tunnel: w7 -> [w28 _ _ w140 _]
    tunnel: "Current source K6221 VISA Device 1" -> [w25 _ _ _ w697]
    tunnel: "Nanovoltmeter 2182a VISA Device1" -> [w24 _ _ _ _]
    tunnel: "Current source K6221 VISA Device 2" -> [w22 _ _ _ w695]
    tunnel: "Nanovoltmeter 2182a VISA Device 2" -> [w21 _ _ _ _]
    tunnel: "Measure two devices?" -> [w16 _ _ _ _]
    tunnel: refnum<visa-resource-name> "COM3" ("GPIB Mercury ITC") -> [_ _ _ w151 w694]
    frame #0 {
      w27 = "Vector Angle (q)"  # Vector Angle (q)
      w15 = "\t"
      n5 = flat-sequence {
        tunnel: w25 -> [w100]
        tunnel: [w98] -> w26
        tunnel: w26 -> [w103]
        tunnel: [w101] -> w23
        tunnel: w24 -> [w105]
        tunnel: w23 -> [w111]
        frame #0 {
          n6 = call "Set-I_K6221_VISA_EL.vi"("Set I (A)"=0.0, "K6221 VISA"=w100) -> ("K6221 VISA out"=w98:refnum<visa-resource-name>)  [unwired: 2 in, 1 out]
        }
        frame #1 {
          n7 = call "KE622x -- Set Output State.vi"("Resource In"=w103, "Output State"=1) -> ("Resource Out (dupl)"=w101:refnum<visa-resource-name>)  [unwired: 12 in, 1 out]
        }
        frame #2 {
          n8 = Wait (ms)(milliseconds to wait=100) -> ()  [unwired: 1 out]
        }
        frame #3 {
          n9 = for {
            N: 5 ("Numeric") -> [_]
            tunnel: w105 -> [w107]
            w109 = u16 1 items=["Slow", "Med", "Fast"] ("Rate (NPLC)")
            w110 = FALSE ("Auto range?")
            n10 = call "Initialize_K2182A_VISA_PK.vi"("VISA address"=w107, "Auto range?"=TRUE, "Analog LPass\nFilter?"=w110, "DC\nFilter?"=w110, "Rate (NPLC)"=w109) -> ()  [unwired: 2 in]
          }
        }
        frame #4 {
          n11 = call "Set-Vcompliance_K6221_VISA_EL.vi"("Set Compliance voltage (V)"="Set Compliance voltage (V)", "K6221 VISA"=w111) -> ()  [unwired: 2 in, 2 out]
        }
      }
      n12 = case shown="True" w16 {
        tunnel: w22 -> [_ w81]
        tunnel: w21 -> [_ w80]
        frame False {
        }
        frame True {
          n13 = flat-sequence {
            tunnel: w81 -> [w85]
            tunnel: [w83] -> w82
            tunnel: w82 -> [w88]
            tunnel: [w86] -> w79
            tunnel: w80 -> [w90]
            tunnel: w79 -> [w96]
            frame #0 {
              n14 = call "Set-I_K6221_VISA_EL.vi"("Set I (A)"=0.0, "K6221 VISA"=w85) -> ("K6221 VISA out"=w83:refnum<visa-resource-name>)  [unwired: 2 in, 1 out]
            }
            frame #1 {
              n15 = call "KE622x -- Set Output State.vi"("Resource In"=w88, "Output State"=1) -> ("Resource Out (dupl)"=w86:refnum<visa-resource-name>)  [unwired: 12 in, 1 out]
            }
            frame #2 {
              n16 = Wait (ms)(milliseconds to wait=100) -> ()  [unwired: 1 out]
            }
            frame #3 {
              n17 = for {
                N: 5 ("Numeric") -> [_]
                tunnel: w90 -> [w92]
                w94 = u16 1 items=["Slow", "Med", "Fast"] ("Rate (NPLC)")
                w95 = FALSE ("Auto range?")
                n18 = call "Initialize_K2182A_VISA_PK.vi"("VISA address"=w92, "Auto range?"=TRUE, "Analog LPass\nFilter?"=w95, "DC\nFilter?"=w95, "Rate (NPLC)"=w94) -> ()  [unwired: 2 in]
              }
            }
            frame #4 {
              n19 = call "Set-Vcompliance_K6221_VISA_EL.vi"("Set Compliance voltage (V)"="Set Compliance voltage (V) 2", "K6221 VISA"=w96) -> ()  [unwired: 2 in, 2 out]
            }
          }
        }
      }
      n20 = case shown="True" w16 {
        tunnel: [FALSE w48] -> w19
        tunnel: "Folder" -> [_ w47]
        frame False {
        }
        frame True {
          w49 = "Vector Angle (q)"  # Vector Angle (q)
          w46 = "\t"
          n21 = Concatenate Strings("File name 2", ".dat" ("string")) -> (w59:string)
          n22 = String To Path(string=w59) -> (path=w53:path)
          n23 = Build Path(base path=w47, name or relative path=w53) -> (appended path=w52:path)
          n24 = Concatenate Strings("Temperature (K)", w46, "Magnetic Field Vector magnitude (T)", w46, w49, w46, "Current (A)" ("string"), w46, "Voltage (V)" ("string"), w46, "Resistance (ohm)" ("string"), w46, "Time (s)", "\r\n") -> (w60:string)
          n25 = flat-sequence {
            tunnel: w52 -> [w68]
            tunnel: w60 -> [w70]
            tunnel: [w70] -> w62
            tunnel: [w69] -> w63
            tunnel: [w64] -> w48
            tunnel: w63 -> [w76]
            tunnel: w62 -> [w77]
            frame #0 {
              n26 = Open/Create/Replace File(file path (use dialog)=w68, operation (0:open)=T1."create") -> (error out=w67:errorcluster)  [unwired: 4 in, 2 out]
              n27 = Unbundle By Name(w67) -> ("status"=w65:bool)
              n28 = case shown="True" w65 {
                tunnel: [FALSE ("Yes") w74] -> w64
                tunnel: [w71 w73] -> w69
                tunnel: w68 -> [w71 w73]
                frame False {
                }
                frame True {
                  n29 = call "Message to User2"() -> ("Yes"=w75:bool)  [unwired: 10 in, 1 out]
                  n30 = Not(x=w75) -> (.not. x?=w74:bool)
                }
              }
            }
            frame #1 {
              n31 = call <vilib>:"Write Characters To File.vi"("append to file? (new file:F)"=TRUE, "character string"=w77, "file path (dialog if empty)"=w76) -> ()  [unwired: 2 in, 1 out]
              "File path 2" <- w76
            }
          }
        }
      }
      n32 = Concatenate Strings("File name 1", ".dat" ("string")) -> (w39:string)
      n33 = String To Path(string=w39) -> (path=w33:path)
      n34 = Build Path(base path="Folder", name or relative path=w33) -> (appended path=w32:path)
      n35 = Concatenate Strings("Temperature (K)", w15, "Magnetic Field Vector magnitude (T)", w15, w27, w15, "Current (A)" ("string"), w15, "Voltage (V)" ("string"), w15, "Resistance (ohm)" ("string"), w15, "Time (s)", "\r\n") -> (w40:string)
      n36 = flat-sequence {
        tunnel: w32 -> [w116]
        tunnel: w40 -> [w119]
        tunnel: [w119] -> w43
        tunnel: [w118] -> w20
        tunnel: [w117] -> w42
        tunnel: w43 -> [w126]
        tunnel: w42 -> [w125]
        tunnel: w31 -> [w129]
        tunnel: w28 -> [w133]
        frame #0 {
          n37 = Open/Create/Replace File(file path (use dialog)=w116, operation (0:open)=T1."create") -> (error out=w115:errorcluster)  [unwired: 4 in, 2 out]
          n38 = Unbundle By Name(w115) -> ("status"=w113:bool)
          n39 = case shown="True" w113 {
            tunnel: [FALSE ("Yes") w123] -> w118
            tunnel: [w120 w122] -> w117
            tunnel: w116 -> [w120 w122]
            frame False {
            }
            frame True {
              n40 = call "Message to User"() -> ("Yes"=w124:bool)  [unwired: 10 in, 1 out]
              n41 = Not(x=w124) -> (.not. x?=w123:bool)
            }
          }
        }
        frame #1 {
          n42 = call <vilib>:"Write Characters To File.vi"("append to file? (new file:F)"=TRUE, "character string"=w126, "file path (dialog if empty)"=w125) -> ()  [unwired: 2 in, 1 out]
          "File path 1" <- w125
        }
        frame #2 {
          n43 = Concatenate Strings("CONFigure:RAMP:RATE:FIELD 1," ("String"), "Sweep Field ramp rate (T/min)", ",3.0") -> (w130:string)
          n44 = call "430_TCP_Command.vi"("Command"=w130, "connection ID"=w129) -> ()  [unwired: 2 in, 3 out]
        }
        frame #3 {
          n45 = Concatenate Strings("CONFigure:RAMP:RATE:FIELD 1," ("String"), "Stable Field ramp rate (T/min)", ",9.0") -> (w135:string)
          n46 = call "430_TCP_Command.vi"("Command"=w135, "connection ID"=w133) -> ()  [unwired: 2 in, 3 out]
        }
      }
      n47 = Or(x=w20, y=w19) -> (x .or. y?=w18:bool)
      n48 = Stop(stop? (T)=w18) -> ()
    }
    frame #1 {
      n49 = flat-sequence {
        frame #0 {
          n50 = Wait (ms)(milliseconds to wait=u32 1000) -> ()  [unwired: 1 out]
        }
      }
    }
    frame #2 {
    }
    frame #3 {
      w145 = u16 1 items=["Off", "31.6 uA", "100 uA", "316 uA", "1.00 mA", "3.16 mA", "10.0 mA", "31.6 mA", "100 mA"] ("Heater Range (0: Off)")
      w146 = u16 2 items=["sample heater", "output 1 (warm-up heater) ", "output 2 (analog/still)"] ("Output (0: sample heater)")
      w155 = u16 0 items=["sample heater", "output 1 (warm-up heater) ", "output 2 (analog/still)"] ("Output (0: sample heater)")
      w154 = u16 0 items=["Unipolar", "Bipolar"] ("Polarity (0: Unipolar)")
      w153 = u16 5 items=["Off", "Monitor Out", "Open Loop (Manual)", "Zone", "Still", "Closed Loop (PID)", "Warm-up"] ("Output Mode (0: Off)")
      w152 = u16 6 items=["1"=1, "2"=2, "3"=3, "4"=4, "5"=5, "6"=6, "7"=7, "8"=8, "9"=9, "10"=10, "11"=11, "12"=12, "13"=13, "14"=14, "15"=15, "16"=16, "A (Control Input)"=17] ("Channel (1:1)")
      w159 = u16 0 items=["none", "1", "2", "3", "4", "5", "6", "7", "8", "9", "10", "11", "12", "13", "14", "15", "16", "A (Control Input)"] ("Channel (1:1)")
      w161 = u16 4 items=["Off"=0, "Monitor Out"=1, "Open Loop (Manual)"=2, "Still"=4] ("Analog Out Mode (0: Off)")
      w162 = u16 2 items=["Kelvin"=1, "Ohms"=2] ("Source (1: Kelvin)")
      n51 = call "Initialize.vi"("Reset (True)"=FALSE, "ID Query (True)"=TRUE, "VISA resource name"=w151) -> ("VISA resource name out"=w156:refnum<visa-resource-name>)  [unwired: 7 in, 1 out]
      n52 = call "Configure Analog Still Output.vi"("VISA resource name"=w156, "Analog Out Mode (0: Off)"=w161, "Source (1: Kelvin)"=w162, "Enable Bipolar Mode (F: Disable)"=FALSE, "Channel (1:1)"=w159, "High Value (0.00000E+0)"=0.0, "Low Value (0.00000E+0)"=0.0, "Manual Value (0.000%)"=0.0, "Still Value (0.000%)"="Still Heater Output (%)") -> ("VISA resource name out"=w143:refnum<visa-resource-name>)  [unwired: 5 in, 1 out]
      n53 = call "Configure Control Parameters.vi"("VISA resource name"=w143, "Output (0: sample heater)"=w146, "Manual Output (0.000%)"=0.0, "Heater Range (0: Off)"=w145) -> ("VISA resource name out"=w142:refnum<visa-resource-name>)  [unwired: 10 in, 1 out]
      n54 = call "Configure Control Mode.vi"("VISA resource name"=w142, "Output (0: sample heater)"=w155, "Channel (1:1)"=w152, "Output Mode (0: Off)"=w153, "Polarity (0: Unipolar)"=w154) -> ("VISA resource name out"=w150:refnum<visa-resource-name>)  [unwired: 9 in, 1 out]
      n55 = for {
        tunnel: w166 -> [w186]
        tunnel: w150 -> [w174]
        tunnel: "From 5" -> [w184] mode=indexing
        tunnel: "Step 5" -> [w183] mode=indexing
        tunnel: "To 5" -> [w182] mode=indexing
        shift-right: [w172] -> _
        shift-left: "Still Heater Output (%)" -> [w173]
        tunnel: w140 -> [w168]
        tunnel: w139 -> [w167]
        w177 = u16 0 items=["none", "1", "2", "3", "4", "5", "6", "7", "8", "9", "10", "11", "12", "13", "14", "15", "16", "A (Control Input)"] ("Channel (1:1)")
        w179 = u16 4 items=["Off"=0, "Monitor Out"=1, "Open Loop (Manual)"=2, "Still"=4] ("Analog Out Mode (0: Off)")
        w180 = u16 2 items=["Kelvin"=1, "Ohms"=2] ("Source (1: Kelvin)")
        n56 = call "Build_serie_EL.vi"("end value"=w182, "increment"=w183, "start value"=w184) -> ("output array"=w185:dbl[])
        n57 = call "Configure Analog Still Output.vi"("VISA resource name"=w174, "Analog Out Mode (0: Off)"=w179, "Source (1: Kelvin)"=w180, "Enable Bipolar Mode (F: Disable)"=FALSE, "Channel (1:1)"=w177, "High Value (0.00000E+0)"=0.0, "Low Value (0.00000E+0)"=0.0, "Manual Value (0.000%)"=0.0, "Still Value (0.000%)"=w173) -> ("VISA resource name out"=w170:refnum<visa-resource-name>)  [unwired: 5 in, 1 out]
        n58 = call "Read Still Output Data.vi"("VISA resource name"=w170) -> ("Heater Output"=→"Still Output (%)":dbl, "VISA resource name out"=w169:refnum<visa-resource-name>)  [unwired: 8 in, 1 out]
        n59 = for {
          tunnel: w186 -> [w194]
          tunnel: w185 -> [w193] mode=indexing
          tunnel: w169 -> [w192]
          tunnel: w168 -> [w188]
          tunnel: w167 -> [w187]
          n60 = flat-sequence {
            tunnel: w194 -> [w202]
            tunnel: [w202] -> w196
            tunnel: w193 -> [w199]
            tunnel: w192 -> [w201]
            tunnel: [w200] -> w191
            tunnel: [w199] -> w190
            tunnel: [w197] -> w189
            tunnel: [w224] -> w195
            tunnel: w196 -> [w224]
            tunnel: w191 -> [w223]
            tunnel: w190 -> [w222]
            tunnel: w189 -> [w221]
            tunnel: w195 -> [w272]
            tunnel: w188 -> [w268]
            tunnel: w187 -> [w267]
            frame #0 {
              n61 = Greater?(x=w199, y=0.0) -> (0:w197:bool)
              n62 = case shown="False" w197 {
                tunnel: w201 -> [w207 w213]
                tunnel: w199 -> [_ w212]
                tunnel: [w206 w209] -> w200
                frame False {
                  w204 = u16 0 items=["Off", "31.6 uA", "100 uA", "316 uA", "1.00 mA", "3.16 mA", "10.0 mA", "31.6 mA", "100 mA"] ("Heater Range (0: Off)")
                  w205 = u16 0 items=["sample heater", "output 1 (warm-up heater) ", "output 2 (analog/still)"] ("Output (0: sample heater)")
                  n63 = call "Configure Control Parameters.vi"("VISA resource name"=w207, "Output (0: sample heater)"=w205, "Manual Output (0.000%)"=0.0, "Heater Range (0: Off)"=w204) -> ("VISA resource name out"=w206:refnum<visa-resource-name>)  [unwired: 10 in, 1 out]
                }
                frame True {
                  n64 = call "T_to_R.vi"("T to convert, K"=w212) -> ("R to set, Ohms"=w215:dbl)  [unwired: 9 in, 1 out]
                  n65 = call "Configure Control Parameters.vi"("VISA resource name"=w213, "Gain(P) (10.000)"="Gain(P) (10.000)", "Reset(I) (20)"="Reset(I) (20)", "Rate(D) (0)"="Rate(D) (0)", "Output (0: sample heater)"="Output (0: sample heater)", "Heater Range (0: Off)"="Heater Range (0: Off)") -> ("VISA resource name out"=w214:refnum<visa-resource-name>)  [unwired: 8 in, 1 out]
                  n66 = call "Configure Setpoint.vi"("Setpoint (0.00000E+0)"=w215, "VISA resource name"=w214) -> ("VISA resource name out"=w208:refnum<visa-resource-name>)  [unwired: 8 in, 1 out]
                  n67 = call "AutoScan.vi"("Autoscan (F: Off)"=FALSE, "Channel (1:1)"=6, "VISA resource name"=w208) -> ("VISA resource name out"=w209:refnum<visa-resource-name>)  [unwired: 7 in, 1 out]
                }
              }
              "Set Temperature (K)" <- w199
            }
            frame #1 {
              n68 = case shown="False" w221 {
                tunnel: w223 -> [w225 w239]
                tunnel: w222 -> [_ w238]
                frame False {
                  n69 = call <vilib>:"High Resolution Relative Seconds.vi"() -> ("relative seconds"=w226:dbl)
                  n70 = while {
                    tunnel: w226 -> [w236]
                    tunnel: w225 -> [w230]
                    stop <- w233 stop-if-true
                    n71 = call <vilib>:"High Resolution Relative Seconds.vi"() -> ("relative seconds"=w237:dbl)
                    n72 = call "Read Sensor Data.vi"("Channel (1:1)"=6, "VISA resource name"=w230) -> ("Kelvin Reading"=w229:dbl)  [unwired: 4 in, 5 out]
                    n73 = local read "T settling delay (s)"() -> (w228:i32)
                    n74 = local write "Current Temperature (K)"(w229) -> ()
                    n75 = Subtract(x=w237, y=w236) -> (x-y=w227:dbl)
                    n76 = local write "Delay timer (s)"(w227) -> ()
                    n77 = Subtract(x=w228, y=w227) -> (x-y=w235:dbl)
                    n78 = Absolute Value(x=w235) -> (abs(x)=w234:dbl)
                    n79 = Less Or Equal?(x=w234, y=0.1) -> (x <= y?=w233:bool)
                  }
                }
                frame True {
                  n80 = flat-sequence {
                    tunnel: w238 -> [w243]
                    tunnel: w239 -> [w242]
                    tunnel: [w241] -> w240
                    tunnel: w240 -> [w254]
                    frame #0 {
                      n81 = while {
                        tunnel: w243 -> [w249]
                        tunnel: w242 -> [w248]
                        tunnel: [w244] -> w241
                        stop <- w251 stop-if-true
                        n82 = call "Read Sensor Data.vi"("Channel (1:1)"=6, "VISA resource name"=w248) -> ("Kelvin Reading"=w245:dbl, "VISA resource name out"=w247:refnum<visa-resource-name>)  [unwired: 4 in, 4 out]
                        "Current Temperature (K)" <- w245
                        n83 = Subtract(x=w245, y=w249) -> (x-y=w250:dbl)
                        n84 = call "Read Still Output Data.vi"("VISA resource name"=w247) -> ("Heater Output"=→"Heater Output (%)":dbl, "VISA resource name out"=w244:refnum<visa-resource-name>)  [unwired: 8 in, 1 out]
                        n85 = Less Or Equal?(x=w250, y=1e-05) -> (x <= y?=w251:bool)
                      }
                    }
                    frame #1 {
                      n86 = call <vilib>:"High Resolution Relative Seconds.vi"() -> ("relative seconds"=w255:dbl)
                      n87 = while {
                        tunnel: w255 -> [w265]
                        tunnel: w254 -> [w257]
                        stop <- w260 stop-if-true
                        n88 = call <vilib>:"High Resolution Relative Seconds.vi"() -> ("relative seconds"=w266:dbl)
                        n89 = call "Read Sensor Data.vi"("Channel (1:1)"=6, "VISA resource name"=w257) -> ("Kelvin Reading"=w256:dbl)  [unwired: 4 in, 5 out]
                        n90 = Subtract(x=w266, y=w265) -> (x-y=w263:dbl)
                        "Delay timer (s)" <- w263
                        n91 = local write "Current Temperature (K)"(w256) -> ()
                        n92 = Subtract(x="T settling delay (s)", y=w263) -> (x-y=w262:dbl)
                        n93 = Absolute Value(x=w262) -> (abs(x)=w261:dbl)
                        n94 = Less Or Equal?(x=w261, y=0.1) -> (x <= y?=w260:bool)
                      }
                    }
                  }
                }
              }
            }
            frame #2 {
              n95 = for {
                tunnel: w272 -> [w279]
                tunnel: "From 2" -> [w278] mode=indexing
                tunnel: "To 2" -> [w277] mode=indexing
                tunnel: "Step 2" -> [w276] mode=indexing
                tunnel: w268 -> [w274]
                tunnel: w267 -> [w273]
                n96 = call "Build_serie_EL.vi"("end value"=w277, "increment"=w276, "start value"=w278) -> ("output array"=w275:dbl[])
                n97 = for {
                  tunnel: w279 -> [w289]
                  tunnel: w275 -> [w282] mode=indexing
                  tunnel: w274 -> [w283]
                  tunnel: w273 -> [w281]
                  n98 = flat-sequence {
                    tunnel: w282 -> [w304]
                    tunnel: w289 -> [w305]
                    tunnel: "Step" -> [w306]
                    tunnel: "To" -> [w307]
                    tunnel: "From" -> [w308]
                    tunnel: [w308] -> w288
                    tunnel: [w307] -> w287
                    tunnel: [w306] -> w286
                    tunnel: [w305] -> w285
                    tunnel: [w304] -> w284
                    tunnel: w283 -> [w300]
                    tunnel: w282 -> [w296]
                    tunnel: [w293] -> w280
                    tunnel: w288 -> [w325]
                    tunnel: w287 -> [w324]
                    tunnel: w286 -> [w323]
                    tunnel: w285 -> [w322]
                    tunnel: w284 -> [w321]
                    tunnel: w281 -> [w320]
                    tunnel: w280 -> [w319]
                    frame #0 {
                      n99 = Number To Fractional String(number=w296) -> (F-format string=w303:string)  [unwired: 3 in]
                      n100 = Concatenate Strings("CONFigure:FIELD:TARGet ", w303) -> (w302:string)
                      n101 = call "430_TCP_Command.vi"("Command"=w302, "connection ID"=w300) -> ("connection ID out"=w298:refnum<k5>)  [unwired: 2 in, 2 out]
                      n102 = call "430_TCP_Command.vi"("Command"="RAMP", "connection ID"=w298) -> ("connection ID out"=w297:refnum<k5>)  [unwired: 2 in, 2 out]
                      n103 = while {
                        tunnel: w297 -> [w316]
                        tunnel: w296 -> [w315]
                        tunnel: [w310] -> w294
                        tunnel: [w309] -> w293
                        stop <- w311 stop-if-true
                        n104 = call "430_TCP_Query.vi"("Command"="FIELD:MAGnet?" ("Magnetic Field (T)"), "connection ID"=w316) -> ("Response"=w317:string, "connection ID out"=w310:refnum<k5>)  [unwired: 5 in, 3 out]
                        n105 = Fract/Exp String To Number(string=w317) -> (number=w309:dbl)  [unwired: 3 in, 1 out]
                        n106 = Subtract(x=w309, y=w315) -> (x-y=w313:dbl)
                        n107 = Absolute Value(x=w313) -> (abs(x)=w314:dbl)
                        n108 = Less Or Equal?(x=w314, y=1e-06) -> (x <= y?=w311:bool)
                      }
                      n109 = call "430_TCP_Command.vi"("Command"="PAUSE", "connection ID"=w294) -> ()  [unwired: 2 in, 3 out]
                    }
                    frame #1 {
                      n110 = for {
                        tunnel: w325 -> [w337] mode=indexing
                        tunnel: w324 -> [w335] mode=indexing
                        tunnel: w323 -> [w336] mode=indexing
                        tunnel: w322 -> [w334]
                        tunnel: w321 -> [w329]
                        tunnel: w320 -> [w327]
                        tunnel: w319 -> [w326]
                        n111 = flat-sequence {
                          tunnel: w334 -> [w339]
                          tunnel: w335 -> [w340]
                          tunnel: w336 -> [w341]
                          tunnel: w337 -> [w342]
                          tunnel: [w342] -> w333
                          tunnel: [w341] -> w332
                          tunnel: [w340] -> w331
                          tunnel: [w339] -> w330
                          tunnel: w329 -> [w338]
                          tunnel: [w338] -> w328
                          tunnel: w333 -> [w350]
                          tunnel: w332 -> [w349]
                          tunnel: w331 -> [w348]
                          tunnel: w330 -> [w346]
                          tunnel: w328 -> [w345]
                          tunnel: w327 -> [w344]
                          tunnel: w326 -> [w343]
                          frame #0 {
                          }
                          frame #1 {
                            n112 = call "Build_serie_EL.vi"("end value"=w348, "increment"=w349, "start value"=w350) -> ("output array"=w347:dbl[])
                            n113 = for {
                              tunnel: w347 -> [w370] mode=indexing
                              tunnel: w346 -> [w369]
                              tunnel: w345 -> [w368]
                              tunnel: w344 -> [w353]
                              tunnel: w343 -> [w351]
                              n114 = flat-sequence {
                                tunnel: w370 -> [w373]
                                tunnel: w368 -> [w381]
                                tunnel: [w381] -> w356
                                tunnel: [w373] -> w355
                                tunnel: [w374] -> w354
                                tunnel: w353 -> [w372]
                                tunnel: [w371] -> w352
                                tunnel: [w392] -> w367
                                tunnel: [w393] -> w366
                                tunnel: w356 -> [_]
                                tunnel: w355 -> [_]
                                tunnel: w354 -> [w394]
                                tunnel: w352 -> [w393]
                                tunnel: w351 -> [w392]
                                tunnel: w367 -> [w401]
                                tunnel: [w401] -> w363
                                tunnel: [w400] -> w365
                                tunnel: w366 -> [w400]
                                tunnel: [w399] -> w361
                                tunnel: [w398] -> w360
                                tunnel: [w397] -> w359
                                tunnel: [w396] -> w358
                                tunnel: w365 -> [w419]
                                tunnel: [w419] -> w364
                                tunnel: w363 -> [w418]
                                tunnel: [w418] -> w362
                                tunnel: w361 -> [w413]
                                tunnel: w360 -> [w412]
                                tunnel: w359 -> [w411]
                                tunnel: w358 -> [w410]
                                tunnel: [w409] -> w357
                                tunnel: w364 -> [w495]
                                tunnel: w362 -> [w489]
                                tunnel: w369 -> [w496]
                                tunnel: w357 -> [w483]
                                frame #0 {
                                n115 = Number To Fractional String(number=w373) -> (F-format string=w375:string)  [unwired: 3 in]
                                n116 = Concatenate Strings("CONFigure:FIELD:TARGet ", w375) -> (w376:string)
                                n117 = call "430_TCP_Command.vi"("Command"=w376, "connection ID"=w372) -> ("connection ID out"=w379:refnum<k5>)  [unwired: 2 in, 2 out]
                                n118 = call "430_TCP_Command.vi"("Command"="RAMP", "connection ID"=w379) -> ("connection ID out"=w380:refnum<k5>)  [unwired: 2 in, 2 out]
                                n119 = while {
                                tunnel: w380 -> [w389]
                                tunnel: w373 -> [w388]
                                tunnel: [w383] -> w374
                                tunnel: [w382] -> w371
                                stop <- w384 stop-if-true
                                n120 = call "430_TCP_Query.vi"("Command"="FIELD:MAGnet?" ("Magnetic Field (T)"), "connection ID"=w389) -> ("Response"=w390:string, "connection ID out"=w383:refnum<k5>)  [unwired: 5 in, 3 out]
                                n121 = Fract/Exp String To Number(string=w390) -> (number=w382:dbl)  [unwired: 3 in, 1 out]
                                n122 = Subtract(x=w382, y=w388) -> (x-y=w386:dbl)
                                n123 = Absolute Value(x=w386) -> (abs(x)=w387:dbl)
                                n124 = Less Or Equal?(x=w387, y=1e-06) -> (x <= y?=w384:bool)
                                }
                                }
                                frame #1 {
                                n125 = call "430_TCP_Command.vi"("Command"="PAUSE", "connection ID"=w394) -> ()  [unwired: 2 in, 3 out]
                                "Stable Magnetic Field magnitude (T)" <- w392
                                "Sweeping Magnetic Field magnitude(T)" <- w393
                                }
                                frame #2 {
                                n126 = local read "Nanovoltmeter 2182a VISA Device 2"() -> (w396:refnum<visa-resource-name>)
                                n127 = local read "Current source K6221 VISA Device 1"() -> (w399:refnum<visa-resource-name>)
                                n128 = local read "Current source K6221 VISA Device 2"() -> (w397:refnum<visa-resource-name>)
                                n129 = local read "Nanovoltmeter 2182a VISA Device1"() -> (w398:refnum<visa-resource-name>)
                                n130 = Multiply(x="Magnetic field stabilization time (s)", y=1000) -> (x*y=w403:dbl)
                                n131 = Wait (ms)(milliseconds to wait=w403) -> ()  [unwired: 1 out]
                                }
                                frame #3 {
                                n132 = flat-sequence {
                                tunnel: w413 -> [w468]
                                tunnel: [w466] -> w417
                                tunnel: w417 -> [w471]
                                tunnel: [w469] -> w416
                                tunnel: w416 -> [w472]
                                tunnel: [w472] -> w415
                                tunnel: w415 -> [w475]
                                tunnel: [w475] -> w414
                                tunnel: w412 -> [w474]
                                tunnel: w414 -> [w481]
                                frame #0 {
                                n133 = call "Set-I_K6221_VISA_EL.vi"("Set I (A)"=0.0, "K6221 VISA"=w468) -> ("K6221 VISA out"=w466:refnum<visa-resource-name>)  [unwired: 2 in, 1 out]
                                }
                                frame #1 {
                                n134 = call "KE622x -- Set Output State.vi"("Resource In"=w471, "Output State"=1) -> ("Resource Out (dupl)"=w469:refnum<visa-resource-name>)  [unwired: 12 in, 1 out]
                                }
                                frame #2 {
                                n135 = Wait (ms)(milliseconds to wait=100) -> ()  [unwired: 1 out]
                                }
                                frame #3 {
                                n136 = for {
                                N: 5 ("Numeric") -> [_]
                                tunnel: w474 -> [w477]
                                w479 = u16 1 items=["Slow", "Med", "Fast"] ("Rate (NPLC)")
                                w480 = FALSE ("Auto range?")
                                n137 = call "Initialize_K2182A_VISA_PK.vi"("VISA address"=w477, "Auto range?"=TRUE, "Analog LPass\nFilter?"=w480, "DC\nFilter?"=w480, "Rate (NPLC)"=w479) -> ()  [unwired: 2 in]
                                }
                                }
                                frame #4 {
                                n138 = local read "Set Compliance voltage (V)"() -> (w482:dbl)
                                n139 = call "Set-Vcompliance_K6221_VISA_EL.vi"("Set Compliance voltage (V)"=w482, "K6221 VISA"=w481) -> ()  [unwired: 2 in, 2 out]
                                }
                                }
                                n140 = local read "Measure two devices?"() -> (w409:bool)
                                n141 = flat-sequence {
                                tunnel: refnum<visa-resource-name> "COM3" ("VISA resource name") -> [w422]
                                tunnel: [w425] -> w408
                                tunnel: w408 -> [w428]
                                tunnel: [w432] -> w407
                                tunnel: w407 -> [w435]
                                tunnel: [w434] -> w405
                                tunnel: w405 -> [w438]
                                frame #0 {
                                n142 = call "AutoScan.vi"("Autoscan (F: Off)"=FALSE, "Channel (1:1)"=3, "VISA resource name"=w422) -> ("VISA resource name out"=w420:refnum<visa-resource-name>)  [unwired: 7 in, 1 out]
                                n143 = call "Read Sensor Data.vi"("Channel (1:1)"=3, "VISA resource name"=w420) -> ("Kelvin Reading"=→"Magnet temperature (K)":dbl, "VISA resource name out"=w425:refnum<visa-resource-name>)  [unwired: 4 in, 4 out]
                                }
                                frame #1 {
                                n144 = call "AutoScan.vi"("Autoscan (F: Off)"=FALSE, "Channel (1:1)"=6, "VISA resource name"=w428) -> ("VISA resource name out"=w427:refnum<visa-resource-name>)  [unwired: 7 in, 1 out]
                                n145 = call "Read Sensor Data.vi"("Channel (1:1)"=6, "VISA resource name"=w427) -> ("Kelvin Reading"=w431:dbl, "VISA resource name out"=w432:refnum<visa-resource-name>)  [unwired: 4 in, 4 out]
                                n146 = local write "Current Temperature (K)"(w431) -> ()
                                }
                                frame #2 {
                                n147 = call "Read Still Output Data.vi"("VISA resource name"=w435) -> ("Heater Output"=w436:dbl, "VISA resource name out"=w434:refnum<visa-resource-name>)  [unwired: 8 in, 1 out]
                                n148 = local write "Heater Output (%)"(w436) -> ()
                                }
                                frame #3 {
                                n149 = call "AutoScan.vi"("Autoscan (F: Off)"=FALSE, "Channel (1:1)"=5, "VISA resource name"=w438) -> ("VISA resource name out"=w439:refnum<visa-resource-name>)  [unwired: 7 in, 1 out]
                                n150 = call "Read Sensor Data.vi"("Channel (1:1)"=5, "VISA resource name"=w439) -> ("Kelvin Reading"=→"Still temperature (K)":dbl)  [unwired: 4 in, 5 out]
                                }
                                }
                                n151 = case shown="True" w409 {
                                tunnel: w411 -> [_ w444]
                                tunnel: w410 -> [_ w443]
                                frame False {
                                }
                                frame True {
                                n152 = flat-sequence {
                                tunnel: w444 -> [w451]
                                tunnel: [w449] -> w448
                                tunnel: w448 -> [w454]
                                tunnel: [w452] -> w447
                                tunnel: w447 -> [w455]
                                tunnel: [w455] -> w446
                                tunnel: w446 -> [w458]
                                tunnel: [w458] -> w445
                                tunnel: w443 -> [w457]
                                tunnel: w445 -> [w464]
                                frame #0 {
                                n153 = call "Set-I_K6221_VISA_EL.vi"("Set I (A)"=0.0, "K6221 VISA"=w451) -> ("K6221 VISA out"=w449:refnum<visa-resource-name>)  [unwired: 2 in, 1 out]
                                }
                                frame #1 {
                                n154 = call "KE622x -- Set Output State.vi"("Resource In"=w454, "Output State"=1) -> ("Resource Out (dupl)"=w452:refnum<visa-resource-name>)  [unwired: 12 in, 1 out]
                                }
                                frame #2 {
                                n155 = Wait (ms)(milliseconds to wait=100) -> ()  [unwired: 1 out]
                                }
                                frame #3 {
                                n156 = for {
                                N: 5 ("Numeric") -> [_]
                                tunnel: w457 -> [w460]
                                w462 = u16 1 items=["Slow", "Med", "Fast"] ("Rate (NPLC)")
                                w463 = FALSE ("Auto range?")
                                n157 = call "Initialize_K2182A_VISA_PK.vi"("VISA address"=w460, "Auto range?"=TRUE, "Analog LPass\nFilter?"=w463, "DC\nFilter?"=w463, "Rate (NPLC)"=w462) -> ()  [unwired: 2 in]
                                }
                                }
                                frame #4 {
                                n158 = local read "Set Compliance voltage (V) 2"() -> (w465:dbl)
                                n159 = call "Set-Vcompliance_K6221_VISA_EL.vi"("Set Compliance voltage (V)"=w465, "K6221 VISA"=w464) -> ()  [unwired: 2 in, 2 out]
                                }
                                }
                                }
                                }
                                }
                                frame #4 {
                                n160 = for {
                                tunnel: w496 -> [w602]
                                tunnel: w489 -> [w600]
                                tunnel: w495 -> [w599]
                                tunnel: "From 3" -> [w594] mode=indexing
                                tunnel: "Step 3" -> [w593] mode=indexing
                                tunnel: "To 3" -> [w592] mode=indexing
                                shift-right: [w591] -> _
                                shift-left: cluster{dbl, "Field Reading":dbl}[] [] -> [w598]
                                shift-right: [w590] -> _
                                shift-left: cluster{dbl, "Field Reading":dbl}[] [] -> [w601]
                                n161 = call "Build_serie_EL.vi"("end value"=w592, "increment"=w593, "start value"=w594) -> ("output array"=w595:dbl[])
                                n162 = local read "Current source K6221 VISA Device 1"() -> (w597:refnum<visa-resource-name>)
                                n163 = local read "Nanovoltmeter 2182a VISA Device1"() -> (w596:refnum<visa-resource-name>)
                                n164 = for {
                                tunnel: w602 -> [w616]
                                tunnel: w600 -> [w610]
                                tunnel: w599 -> [w609]
                                tunnel: w595 -> [w607] mode=indexing
                                shift-right: [w603] -> w590
                                shift-left: w601 -> [w615]
                                shift-right: [w604] -> w591
                                shift-left: w598 -> [w608]
                                tunnel: w597 -> [w606]
                                tunnel: w596 -> [w605]
                                n165 = Tick Count (ms)() -> (millisecond timer value=w612:u32)
                                n166 = Subtract(x=w612, y=w616) -> (x-y=w614:u32)
                                n167 = Divide(x=w614, y=1000.0) -> (x/y=w611:dbl)
                                "Time (s)" <- w611
                                n168 = stacked-sequence {
                                tunnel: w615 -> [_ w638 _ _]
                                tunnel: [_ w639 _ _] -> w603
                                tunnel: w611 -> [_ w626 _ _]
                                tunnel: w610 -> [_ w633 _ _]
                                tunnel: w609 -> [_ w632 _ _]
                                tunnel: [_ w631 _ _] -> w604
                                tunnel: w608 -> [_ w629 _ _]
                                tunnel: w607 -> [w618 _ _ _]
                                tunnel: w606 -> [w617 w623 _ _]
                                tunnel: w605 -> [_ w622 _ _]
                                frame #0 {
                                n169 = flat-sequence {
                                tunnel: w618 -> [w620]
                                tunnel: w617 -> [w619]
                                frame #0 {
                                n170 = call "Set-I_K6221_VISA_EL.vi"("Set I (A)"=w620, "K6221 VISA"=w619) -> ()  [unwired: 2 in, 2 out]
                                }
                                frame #1 {
                                n171 = Wait (ms)(milliseconds to wait="wait (ms)") -> ()  [unwired: 1 out]
                                }
                                }
                                }
                                frame #1 {
                                n172 = flat-sequence {
                                tunnel: [w644] -> w637
                                tunnel: [w650] -> w636
                                tunnel: [w646] -> w635
                                tunnel: [w649] -> w634
                                tunnel: [w648] -> w630
                                tunnel: "Number Averaging" -> [w643]
                                tunnel: w629 -> [w648]
                                tunnel: w638 -> [w650]
                                tunnel: w633 -> [w649]
                                tunnel: [w644] -> w627
                                tunnel: [w646] -> w625
                                tunnel: [w647] -> w624
                                tunnel: w623 -> [w641]
                                tunnel: w622 -> [w640]
                                tunnel: w637 -> [w673]
                                tunnel: [w683] -> w639
                                tunnel: w636 -> [w682]
                                tunnel: w635 -> [w672]
                                tunnel: w634 -> [w677]
                                tunnel: w626 -> [w680]
                                tunnel: w632 -> [w679]
                                tunnel: [w675] -> w631
                                tunnel: w630 -> [w674]
                                tunnel: w627 -> [w676]
                                tunnel: w626 -> [w671]
                                tunnel: w625 -> [w670]
                                tunnel: w624 -> [w669]
                                frame #0 {
                                n173 = for {
                                N: w643 -> [_]
                                tunnel: [w652] -> w642 mode=indexing
                                tunnel: [w651] -> w645 mode=indexing
                                tunnel: w641 -> [w657]
                                tunnel: w640 -> [w658]
                                n174 = flat-sequence {
                                tunnel: w657 -> [w659]
                                tunnel: w658 -> [w661]
                                tunnel: [w661] -> w656
                                tunnel: [w660] -> w655
                                tunnel: w656 -> [w664]
                                tunnel: w655 -> [w663]
                                tunnel: [w664] -> w654
                                tunnel: [w663] -> w653
                                tunnel: [w667] -> w651
                                tunnel: w654 -> [w666]
                                tunnel: w653 -> [w667]
                                tunnel: [w665] -> w652
                                frame #0 {
                                n175 = call "KE622x -- Get Current Level.vi"("Resource In"=w659) -> ("Current Level (A)"=w660:T2)  [unwired: 12 in, 2 out]
                                }
                                frame #1 {
                                n176 = Wait (ms)(milliseconds to wait=50) -> ()  [unwired: 1 out]
                                }
                                frame #2 {
                                n177 = call "Get-V_K2182A_VISA_EL.vi"("VISA K2182A"=w666) -> ("V (V)"=w665:dbl)  [unwired: 2 in, 2 out]
                                }
                                }
                                }
                                n178 = call "Array averaging_PK.vi"("Number averaging"=w643, "numeric array"=w645) -> ("Average value"=w646:dbl)  [unwired: 9 in]
                                "Iset (A)" <- w646
                                n179 = call "Array averaging_PK.vi"("Number averaging"=w643, "numeric array"=w642) -> ("Average value"=w644:dbl)  [unwired: 9 in]
                                "Vmeas (V)" <- w644
                                n180 = Divide(x=w644, y=w646) -> (x/y=w647:dbl)
                                "Resistance (ohm)" <- w647
                                }
                                frame #1 {
                                n181 = Bundle(w671, "Average value"=w676) -> (w678:cluster{dbl, "Average value":dbl})  [unwired: 1 in]
                                n182 = Bundle("Average value"=w670, "Average value"=w676) -> (w681:T3)  [unwired: 1 in]
                                n183 = local read "Current Temperature (K)"() -> (w668:dbl)
                                n184 = Build Array (concatenate)(w674, w678) -> (w675:cluster{dbl, "Average value":dbl}[])
                                n185 = Build Array (concatenate)(w682, w681) -> (w683:T4)
                                "V vs I" <- w683
                                n186 = Build Array(w668, w677, w679, w672, w673, w669, w680) -> (→"data":dbl[])
                                }
                                }
                                }
                                frame #2 {
                                n187 = Wait (ms)(milliseconds to wait=u32 50) -> ()  [unwired: 1 out]
                                }
                                frame #3 {
                                n188 = local read "data"() -> (w686:dbl[])
                                n189 = Array To Spreadsheet String(array=w686, 3:"%e" ("format string")) -> (spreadsheet string=w689:string)  [unwired: 1 in]
                                n190 = local read "File path 1"() -> (w688:path)
                                n191 = call <vilib>:"Write Characters To File.vi"("append to file? (new file:F)"=TRUE, "character string"=w689, "file path (dialog if empty)"=w688) -> ()  [unwired: 2 in, 1 out]
                                }
                                }
                                }
                                }
                                n192 = case shown="True" w483 {
                                tunnel: "From 4" -> [_ w501]
                                tunnel: "To 4" -> [_ w500]
                                tunnel: "Step 4" -> [_ w499]
                                tunnel: cluster{dbl, "Field Reading":dbl}[] [] -> [_ w498]
                                tunnel: cluster{dbl, "Field Reading":dbl}[] [] -> [_ w497]
                                frame False {
                                }
                                frame True {
                                n193 = for {
                                tunnel: w501 -> [w508] mode=indexing
                                tunnel: w500 -> [w507] mode=indexing
                                tunnel: w499 -> [w506] mode=indexing
                                shift-right: [w503] -> _
                                shift-left: w498 -> [w505]
                                shift-right: [w502] -> _
                                shift-left: w497 -> [w504]
                                n194 = call "Build_serie_EL.vi"("end value"=w507, "increment"=w506, "start value"=w508) -> ("output array"=w509:dbl[])
                                n195 = local read "Nanovoltmeter 2182a VISA Device 2"() -> (w510:refnum<visa-resource-name>)
                                n196 = local read "Current source K6221 VISA Device 2"() -> (w511:refnum<visa-resource-name>)
                                n197 = for {
                                tunnel: w509 -> [w517] mode=indexing
                                shift-right: [w513] -> w502
                                shift-left: w504 -> [w519]
                                shift-right: [w514] -> w503
                                shift-left: w505 -> [w518]
                                tunnel: w511 -> [w516]
                                tunnel: w510 -> [w515]
                                n198 = local read "Time (s)"() -> (w512:dbl)
                                n199 = stacked-sequence {
                                tunnel: w519 -> [_ w538 _ _]
                                tunnel: [_ w539 _ _] -> w513
                                tunnel: w512 -> [_ w530 _ _]
                                tunnel: [_ w534 _ _] -> w514
                                tunnel: w518 -> [_ w532 _ _]
                                tunnel: w517 -> [w521 _ _ _]
                                tunnel: w516 -> [w520 w527 _ _]
                                tunnel: w515 -> [_ w526 _ _]
                                frame #0 {
                                n200 = flat-sequence {
                                tunnel: w521 -> [w523]
                                tunnel: w520 -> [w522]
                                frame #0 {
                                n201 = call "Set-I_K6221_VISA_EL.vi"("Set I (A)"=w523, "K6221 VISA"=w522) -> ()  [unwired: 2 in, 2 out]
                                }
                                frame #1 {
                                n202 = Wait (ms)(milliseconds to wait="wait (ms) 2") -> ()  [unwired: 1 out]
                                }
                                }
                                }
                                frame #1 {
                                n203 = local read "Number Averaging"() -> (w525:i32)
                                n204 = flat-sequence {
                                tunnel: [w544] -> w537
                                tunnel: [w549] -> w536
                                tunnel: [w546] -> w535
                                tunnel: [w548] -> w533
                                tunnel: w525 -> [w543]
                                tunnel: w532 -> [w548]
                                tunnel: w538 -> [w549]
                                tunnel: [w544] -> w531
                                tunnel: [w546] -> w529
                                tunnel: [w547] -> w528
                                tunnel: w527 -> [w541]
                                tunnel: w526 -> [w540]
                                tunnel: w537 -> [w574]
                                tunnel: [w582] -> w539
                                tunnel: w536 -> [w581]
                                tunnel: w535 -> [w573]
                                tunnel: w530 -> [w579]
                                tunnel: [w576] -> w534
                                tunnel: w533 -> [w575]
                                tunnel: w531 -> [w577]
                                tunnel: w530 -> [w572]
                                tunnel: w529 -> [w571]
                                tunnel: w528 -> [w570]
                                frame #0 {
                                n205 = for {
                                N: w543 -> [_]
                                tunnel: [w551] -> w542 mode=indexing
                                tunnel: [w550] -> w545 mode=indexing
                                tunnel: w541 -> [w556]
                                tunnel: w540 -> [w557]
                                n206 = flat-sequence {
                                tunnel: w556 -> [w558]
                                tunnel: w557 -> [w560]
                                tunnel: [w560] -> w555
                                tunnel: [w559] -> w554
                                tunnel: w555 -> [w563]
                                tunnel: w554 -> [w562]
                                tunnel: [w563] -> w553
                                tunnel: [w562] -> w552
                                tunnel: [w566] -> w550
                                tunnel: w553 -> [w565]
                                tunnel: w552 -> [w566]
                                tunnel: [w564] -> w551
                                frame #0 {
                                n207 = call "KE622x -- Get Current Level.vi"("Resource In"=w558) -> ("Current Level (A)"=w559:T2)  [unwired: 12 in, 2 out]
                                }
                                frame #1 {
                                n208 = Wait (ms)(milliseconds to wait=50) -> ()  [unwired: 1 out]
                                }
                                frame #2 {
                                n209 = call "Get-V_K2182A_VISA_EL.vi"("VISA K2182A"=w565) -> ("V (V)"=w564:dbl)  [unwired: 2 in, 2 out]
                                }
                                }
                                }
                                n210 = call "Array averaging_PK.vi"("Number averaging"=w543, "numeric array"=w542) -> ("Average value"=w544:dbl)  [unwired: 9 in]
                                "Vmeas (V) 2" <- w544
                                n211 = call "Array averaging_PK.vi"("Number averaging"=w543, "numeric array"=w545) -> ("Average value"=w546:dbl)  [unwired: 9 in]
                                "Iset (A) 2" <- w546
                                n212 = Divide(x=w544, y=w546) -> (x/y=w547:dbl)
                                "Resistance (ohm) 2" <- w547
                                }
                                frame #1 {
                                n213 = Bundle("Time (s)"=w572, "Average value"=w577) -> (w578:cluster{"Time (s)":dbl, "Average value":dbl})  [unwired: 1 in]
                                n214 = Bundle("Average value"=w571, "Average value"=w577) -> (w580:T3)  [unwired: 1 in]
                                n215 = Build Array (concatenate)(w575, w578) -> (w576:cluster{"Time (s)":dbl, "Average value":dbl}[])
                                n216 = Build Array (concatenate)(w581, w580) -> (w582:T4)
                                "V vs I 2" <- w582
                                n217 = local read "Sweeping Magnetic Field magnitude(T)"() -> (w568:dbl)
                                n218 = local read "Stable Magnetic Field magnitude (T)"() -> (w569:dbl)
                                n219 = local read "Current Temperature (K)"() -> (w567:dbl)
                                n220 = Build Array(w567, w569, w568, w573, w574, w570, w579) -> (→"data 2":dbl[])
                                }
                                }
                                }
                                frame #2 {
                                n221 = Wait (ms)(milliseconds to wait=u32 50) -> ()  [unwired: 1 out]
                                }
                                frame #3 {
                                n222 = local read "data 2"() -> (w585:dbl[])
                                n223 = local read "File path 2"() -> (w587:path)
                                n224 = Array To Spreadsheet String(array=w585, 3:"%e" ("format string")) -> (spreadsheet string=w588:string)  [unwired: 1 in]
                                n225 = call <vilib>:"Write Characters To File.vi"("append to file? (new file:F)"=TRUE, "character string"=w588, "file path (dialog if empty)"=w587) -> ()  [unwired: 2 in, 1 out]
                                }
                                }
                                }
                                }
                                }
                                }
                                }
                              }
                            }
                          }
                          frame #2 {
                            n226 = Multiply(x="Wait time after each sweep(min)", y=60000.0) -> (x*y=w693:dbl)
                            n227 = Wait (ms)(milliseconds to wait=w693) -> ()  [unwired: 1 out]
                          }
                        }
                      }
                    }
                  }
                }
              }
            }
          }
        }
        n228 = local read "Still Heater Output (%)"() -> (w172:dbl)
      }
    }
    frame #4 {
      n229 = flat-sequence {
        tunnel: w697 -> [w706]
        tunnel: [w704] -> w698
        tunnel: w698 -> [w708]
        frame #0 {
          n230 = call "Set-I_K6221_VISA_EL.vi"("Set I (A)"=0.0, "K6221 VISA"=w706) -> ("K6221 VISA out"=w704:refnum<visa-resource-name>)  [unwired: 2 in, 1 out]
        }
        frame #1 {
          n231 = call "KE622x -- Set Output State.vi"("Resource In"=w708, "Output State"=0) -> ()  [unwired: 12 in, 2 out]
        }
      }
      n232 = flat-sequence {
        tunnel: w695 -> [w701]
        tunnel: [w699] -> w696
        tunnel: w696 -> [w703]
        frame #0 {
          n233 = call "Set-I_K6221_VISA_EL.vi"("Set I (A)"=0.0, "K6221 VISA"=w701) -> ("K6221 VISA out"=w699:refnum<visa-resource-name>)  [unwired: 2 in, 1 out]
        }
        frame #1 {
          n234 = call "KE622x -- Set Output State.vi"("Resource In"=w703, "Output State"=0) -> ()  [unwired: 12 in, 2 out]
        }
      }
      n235 = call "Close.vi"("VISA resource name"=w694) -> ()  [unwired: 10 in, 1 out]
    }
  }
